vi "WS1050 36 DUT Characterization Ver1.0.vi"() -> ()   [LabVIEW 2012]
uses:
  WS_VCAP Driver 029/Source/WSVCAP Shell/Type Defs/WSVCAP SHL I2C DUT Mask Mode Enum.ctl
  <vilib>/Utility/file.llb/Read From Spreadsheet File (DBL).vi
panel:
  out "VISA resource name out":refnum<visa-resource-name>="GPIB0::3::INSTR"
  out "error out 2":errorcluster={"status"=TRUE, "code"=-63192, "source"="niLvFpga_Open_PXI-7813R.vi"}
  in  "Reg1_Bit Cntrl":string[](array[string])=["01", "02", "04", "08", "10", "20", "40", "80", "03", "06", "0C", "D8", "33", "66", "CC", "07", "0E", "1C", "38", "70", "E0", "0F", "1E", "3C", "78", "F0", "1F", "3E", "7C", "F8", "3F", "7E", "FC", "7F", "FE", "FD", "FB", "F7", "EF", "DF", "BF", "7F", "FC", "F9", "F3", "E7", "CF", "9F", "3F", "F8", "F1", "E3", "C7", "8F", "1F", "F0", "E1", "C3", "87", "0F", "E0", "C1", "83", "07", "C0", "81", "03", "AA", "55", "00"]
  out "date string":string="5/19/2014"
  out "PS1 Out":refnum<visa-resource-name>
  out "Ke2000 Out":refnum<visa-resource-name>="GPIB0::9::INSTR"
  in  "VPI_Cmd":string[](array[string])=["00", "3B", "00"]
  in  "VPI Name":string[](array[string])=["All_Drivers OFF", "All Drivers ON", "All Drivers OFF2"]
  in  "Tab Control":T1(tab)
  in  "No of Cmd":i64=3
  in  "Board#":string="BRD5"
  in  "Serial Number":string[][](table)=[["DUT", "SN"], ["DUT1", "1"], ["DUT2", "2"], ["DUT3", "3"], ["DUT4", "4"], ["DUT5", "5"], ["DUT6", "6"], ["DUT7", "7"], ["DUT8", "8"], ["DUT9", "9"], ["DUT10", "10"], ["DUT11", "11"], ["DUT12", "12"], ["DUT13", "13"], ["DUT14", "14"], ["DUT15", "15"], ["DUT16", "16"], ["DUT17", "17"], ["DUT18", "18"], ["DUT19", "19"], ["DUT20", "20"], ["DUT21", "21"], ["DUT22", "22"], ["DUT23", "23"], ["DUT24", "24"], ["DUT25", "25"], ["DUT26", "26"], ["DUT27", "27"], ["DUT28", "28"], ["DUT29", "29"], ["DUT30", "30"], ["DUT31", "31"], ["DUT32", "32"], ["DUT33", "33"], ["DUT34", "34"], ["DUT35", "35"], ["DUT36", "36"]]
  in  "SPI Clock Rate (Hz)":dbl=5000000.0 caption="Cycle Speed" format="%.1p Hz"
  in  "Wafer#":string="T7-EB"
  in  "File Name":string="CYC_WS1050_T7_EB_65C_40V_25DC_EMPTY_BRD5_141017_1"
  in  "TMN DC\\CAP Data Log File Path":path=path "C:/WS1050 36 DUT Data"
  in  "Test Program":string="WS1050 36 DUT Characterization Ver1.0"
  out "Current Date":string="8/28/2014"
  out "Current Time":string="0950"
  in  "Start Date":string="10/21/2014"
  in  "Start Time":string="1542"
  in  "Comment":string="CYC65C40V"
  in  "OK Button":bool
  in  "Calibration":bool
  in  "Verify CP":bool
  in  "CP Setting":i32(ring) items=["CP OFF", "CP ON", "CP 35V", "CP 40V", "DVA ON", "DVA OFF", "REG1 ON", "REG1 OFF", "REG2 ON", "REG2 OFF", "REG3 ON", "REG3 OFF"]
  in  "Stop Calibration":bool
  in  "Set VDD":dbl=3.3 format="%.3g"
  in  "Command":string[](array[string])=["07020100003B", "070201003B00", "0702013B0000"]
  in  "Clock Rate (Hz)":dbl=1000000.0 caption="Meas Speed" format="%.1p Hz"
  out "AR  Measurent(Hz)":dbl
  in  "PS1 Source":refnum<visa-resource-name>="GPIB0::5::INSTR"
  in  "Ke2000":refnum<visa-resource-name>="GPIB0::9::INSTR"
  in  "Set CP to Meas":i32(ring) items=["CP OFF", "CP 23.75V ", "CP 24.5V", "CP 25.25V", "CP 26V", "CP 26.75V", "CP 27.5V", "CP 28.25V", "CP 29V", "CP 29.75V", "CP 30.5V", "CP 31.25V", "CP 32V", "CP 32.75V", "CP 33.5V", "CP 34.25V", "CP 35V", "CP 35.75V", "CP 36.5V", "CP 37.25V", "CP 38V", "CP 38.75V", "CP 39.5V", "CP 40.25V", "CP 41V", "CP 41.75V", "CP 42.5V", "CP 43.25V", "CP 44V", "CP 50V", "CP 55V"]
  out "Simulate FPGA":bool
  out "Online":bool
  out "AR Cycling(Hz)":dbl=5000000.0
  in  "Ke2400":refnum<visa-resource-name>="GPIB0::3::INSTR"
  in  "Initialize AD7747":bool
  in  "DUT Mask Mode":T2=enum."All"
  in  "RFFE Slave Address":u8=7 caption="Slave Address" format="0x%02x"
  out "Activity Log":string="05/19/2014 -- 12:24:35.853::WSVCAP::APP::Application Started\n05/19/2014 -- 12:24:37.606::WSVCAP::WSVCAP SHL::WR I2C-REG:0x0A;MASK:0xFFFFFFFFFFFF;C1 DATA:22:22:22:22:22:22:22:22:22:22:22:22:22:22:22:22;C2 DATA:22:22:22:22:22:22:22:22:22:22:22:22:22:22:22:22;C3 DATA:22:22:22:22:22:22:22:22:22:22:22:22:22:22:22:22\r\n05/19/2014 -- 12:24:37.773::WSVCAP::WSVCAP SHL::WR I2C-ST:0,0,4,1\r\n05/19/2014 -- 12:24:37.903::WSVCAP::WSVCAP SHL::RD I2C-BYTES:4;ADD:0x00;MASK:0xFFFFFFFFFFFF\r\n05/19/2014 -- 12:24:38.045::WSVCAP::WSVCAP SHL::RD I2C:C1 DATA:2:2:2:2:2:2:2:2:2:2:2:2:2:2:2:2|A7:A9:AA:82:82:7F:82:81:82:81:83:82:81:82:82:81|46:36:BB:88:44:A3:E9:2B:32:20:ED:25:BB:3D:68:B|2C:6A:EB:A7:22:56:FE:CC:36:82:D7:B0:3B:48:F9:CC;C2 DATA:2:2:2:2:2:2:2:2:2:2:2:2:2:2:2:2|94:94:94:80:80:80:80:80:81:7E:7E:81:80:7E:80:80|47:33:15:82:62:B:E8:1C:D7:C3:7D:41:7C:B7:4C:2A|C4:B4:AE:8:1E:D1:4E:37:11:C0:6F:63:42:9D:63:B5;C3 DATA:2:2:2:2:2:2:2:2:2:2:2:2:2:2:2:2|95:95:95:81:81:7E:81:80:84:7D:80:83:81:7E:7F:80|AB:C4:14:B5:7B:52:DF:C9:79:5D:5F:30:99:31:1E:F4|6E:5C:F7:A8:C3:EB:7B:EF:33:92:89:77:4D:67:75:DD;STATUS:0:0:4:0\r\n05/19/2014 -- 12:24:38.046::WSVCAP::WSVCAP SHL::WR I2C-REG:0x0A;MASK:0xFFFFFFFFFFFF;C1 DATA:22:22:22:22:22:22:22:22:22:22:22:22:22:22:22:22;C2 DATA:22:22:22:22:22:22:22:22:22:22:22:22:22:22:22:22;C3 DATA:22:22:22:22:22:22:22:22:22:22:22:22:22:22:22:22\r\n05/19/2014 -- 12:24:38.089::WSVCAP::WSVCAP SHL::WR I2C-ST:0,0,4,1\r\n05/19/2014 -- 12:24:38.219::WSVCAP::WSVCAP SHL::RD I2C-BYTES:4;ADD:0x00;MASK:0xFFFFFFFFFFFF\r\n05/19/2014 -- 12:24:38.362::WSVCAP::WSVCAP SHL::RD I2C:C1 DATA:2:2:2:2:2:2:2:2:2:2:2:2:2:2:2:2|A7:AB:AA:82:82:82:83:83:82:82:82:82:7F:82:82:81|4B:32:96:83:3E:61:43:17:25:62:AB:4D:A2:40:2E:5|3C:76:2B:B4:EE:E4:A9:1A:AA:A:26:C7:21:2E:87:5B;C2 DATA:2:2:2:2:2:2:2:2:2:2:2:2:2:2:2:2|94:94:94:80:80:80:80:80:80:7F:80:81:80:80:7F:80|4A:32:19:7D:19:6C:79:46:61:7F:4B:B8:A5:30:F3:14|B4:70:A:8C:9C:DC:43:FA:1E:A:C6:21:A:A9:13:F3;C3 DATA:2:2:2:2:2:2:2:2:2:2:2:2:2:2:2:2|95:97:94:81:80:81:82:81:80:7E:81:84:7F:81:80:80|B2:32:D0:A7:9E:4C:AB:D4:EE:D9:F0:82:B7:91:7:FF|C1:91:B6:3D:D8:E:1B:4F:9F:6A:F1:6C:E7:3F:7:BA;STATUS:0:0:4:0\r\n05/19/2014 -- 12:24:38.364::WSVCAP::WSVCAP SHL::WR I2C-REG:0x0A;MASK:0xFFFFFFFFFFFF;C1 DATA:22:22:22:22:22:22:22:22:22:22:22:22:22:22:22:22;C2 DATA:22:22:22:22:22:22:22:22:22:22:22:22:22:22:22:22;C3 DATA:22:22:22:22:22:22:22:22:22:22:22:22:22:22:22:22\r\n05/19/2014 -- 12:24:38.406::WSVCAP::WSVCAP SHL::WR I2C-ST:0,0,4,1\r\n05/19/2014 -- 12:24:38.536::WSVCAP::WSVCAP SHL::RD I2C-BYTES:4;ADD:0x00;MASK:0xFFFFFFFFFFFF\r\n05/19/2014 -- 12:24:38.678::WSVCAP::WSVCAP SHL::RD I2C:C1 DATA:2:2:2:2:2:2:2:2:2:2:2:2:2:2:2:2|A7:A9:AB:82:82:81:82:82:82:82:82:82:82:82:82:81|46:71:4C:87:43:3D:7F:FC:25:4F:8E:54:97:3E:60:8C|AA:F4:1F:B5:CE:43:1F:36:9:87:9C:78:86:5:B6:8E;C2 DATA:2:2:2:2:2:2:2:2:2:2:2:2:2:2:2:2|94:94:94:80:7F:7F:80:80:80:80:80:81:80:80:80:80|49:36:18:7D:6E:C5:E4:3C:81:2E:41:D3:75:71:E3:72|E8:D3:E6:D1:E0:48:AE:D4:54:D:E8:8E:B4:41:68:4;C3 DATA:2:2:2:2:2:2:2:2:2:2:2:2:2:2:2:2|95:95:95:81:7F:7F:81:81:81:81:81:84:81:81:82:81|B3:F5:90:AB:82:69:7B:93:D0:77:E8:D5:E8:8C:84:E8|B9:AC:EE:2B:B6:71:8F:4A:74:31:56:BB:8A:B7:A0:C8;STATUS:0:0:4:0\r\n05/19/2014 -- 12:24:38.681::WSVCAP::WSVCAP SHL::WR I2C-REG:0x0A;MASK:0xFFFFFFFFFFFF;C1 DATA:22:22:22:22:22:22:22:22:22:22:22:22:22:22:22:22;C2 DATA:22:22:22:22:22:22:22:22:22:22:22:22:22:22:22:22;C3 DATA:22:22:22:22:22:22:22:22:22:22:22:22:22:22:22:22\r\n05/19/2014 -- 12:24:38.723::WSVCAP::WSVCAP SHL::WR I2C-ST:0,0,4,1\r\n05/19/2014 -- 12:24:38.854::WSVCAP::WSVCAP SHL::RD I2C-BYTES:4;ADD:0x00;MASK:0xFFFFFFFFFFFF\r\n05/19/2014 -- 12:24:38.996::WSVCAP::WSVCAP SHL::RD I2C:C1 DATA:2:2:2:2:2:2:2:2:2:2:2:2:2:2:2:2|A7:A9:AA:82:82:7F:83:81:82:81:84:82:7F:82:7F:82|43:FB:E:7F:3C:AD:35:35:26:A2:6C:21:4B:3D:8:6|63:9A:E1:F3:95:32:91:42:90:3C:78:1F:5C:D7:5F:D8;C2 DATA:2:2:2:2:2:2:2:2:2:2:2:2:2:2:2:2|94:94:94:80:80:80:80:80:81:80:7E:81:80:7E:7F:80|48:36:18:7F:5E:3D:69:83:DE:AE:A1:9E:31:AE:BB:96|15:A0:44:17:13:FD:CC:C8:6D:B2:EF:A7:C:C7:3B:F;C3 DATA:2:2:2:2:2:2:2:2:2:2:2:2:2:2:2:2|95:96:94:81:81:7E:82:80:84:80:80:84:7F:7E:7D:82|AD:3B:6D:A9:7C:57:9D:F5:7A:96:23:5C:36:2D:ED:5A|CD:46:DB:3B:C7:BD:70:60:33:B8:B:F7:63:A:51:4D;STATUS:0:0:4:0\r\n05/19/2014 -- 12:24:38.998::WSVCAP::WSVCAP SHL::WR I2C-REG:0x0A;MASK:0xFFFFFFFFFFFF;C1 DATA:22:22:22:22:22:22:22:22:22:22:22:22:22:22:22:22;C2 DATA:22:22:22:22:22:22:22:22:22:22:22:22:22:22:22:22;C3 DATA:22:22:22:22:22:22:22:22:22:22:22:22:22:22:22:22\r\n05/19/2014 -- 12:24:39.040::WSVCAP::WSVCAP SHL::WR I2C-ST:0,0,4,1\r\n05/19/2014 -- 12:24:39.170::WSVCAP::WSVCAP SHL::RD I2C-BYTES:4;ADD:0x00;MASK:0xFFFFFFFFFFFF\r\n05/19/2014 -- 12:24:39.311::WSVCAP::WSVCAP SHL::RD I2C:C1 DATA:2:2:2:2:2:2:2:2:2:2:2:2:2:2:2:2|A7:AA:AB:82:82:81:82:81:82:81:82:82:82:82:7F:82|44:F1:90:87:45:44:C8:2C:2C:F1:FC:1B:94:3B:3C:75|4A:49:95:19:99:73:64:3:23:24:F3:A2:5E:7F:C4:B6;C2 DATA:2:2:2:2:2:2:2:2:2:2:2:2:2:2:2:2|94:94:94:80:80:80:80:7F:80:80:7E:80:80:7E:7F:80|4C:36:17:7D:A8:9F:DE:C7:53:6D:8A:F4:41:A5:C6:E0|90:2E:24:C:D9:22:E4:76:3B:40:1D:53:33:B1:3E:4D;C3 DATA:2:2:2:2:2:2:2:2:2:2:2:2:2:2:2:2|95:97:95:81:81:7F:81:80:80:81:7F:82:81:7E:7D:82|AE:2B:A7:AB:CC:CD:A4:38:FD:17:80:F2:92:2D:45:C4|76:E5:D:B9:AD:B5:BA:8D:28:32:9E:42:B7:20:4A:D9;STATUS:0:0:4:0\r\n05/19/2014 -- 12:24:39.313::WSVCAP::WSVCAP SHL::WR I2C-REG:0x0A;MASK:0xFFFFFFFFFFFF;C1 DATA:22:22:22:22:22:22:22:22:22:22:22:22:22:22:22:22;C2 DATA:22:22:22:22:22:22:22:22:22:22:22:22:22:22:22:22;C3 DATA:22:22:22:22:22:22:22:22:22:22:22:22:22:22:22:22\r\n05/19/2014 -- 12:24:39.355::WSVCAP::WSVCAP SHL::WR I2C-ST:0,0,4,1\r\n05/19/2014 -- 12:24:39.486::WSVCAP::WSVCAP SHL::RD I2C-BYTES:4;ADD:0x00;MASK:0xFFFFFFFFFFFF\r\n05/19/2014 -- 12:24:39.628::WSVCAP::WSVCAP SHL::RD I2C:C1 DATA:2:2:2:2:2:2:2:2:2:2:2:2:2:2:2:2|A7:A9:AA:82:82:82:83:82:82:82:82:82:7F:82:7F:82|47:18:E4:87:3E:E7:6:65:25:92:37:38:A8:3E:89:85|7C:A7:7:2B:A3:7A:EC:EF:89:ED:F4:D3:D8:BC:3A:F5;C2 DATA:2:2:2:2:2:2:2:2:2:2:2:2:2:2:2:2|94:94:94:80:7F:80:80:7F:81:80:7E:80:80:80:81:80|49:37:17:80:76:25:6A:F8:DF:55:97:4D:B8:5B:2B:B1|13:E3:9A:3E:1A:2D:4F:B6:DB:E9:61:FA:8B:D6:9:CC;C3 DATA:2:2:2:2:2:2:2:2:2:2:2:2:2:2:2:2|95:95:95:81:7F:80:82:81:84:80:7F:81:80:81:7F:82|AF:93:3B:AF:5B:11:82:E4:7E:C3:2D:72:9:96:D9:A|DB:96:F2:10:5F:64:9A:C6:98:12:27:7D:10:D3:20:D9;STATUS:0:0:4:0\r\n05/19/2014 -- 12:24:40.132::WSVCAP::WSVCAP SHL::CLOSE\r\n"
  in  "C1 Cap DAC":u8=128 caption="B Data In" format="0x%02x"
  in  "C2 Cap DAC":u8=128 caption="B Data In" format="0x%02x"
  in  "C3 Cap DAC":u8=128 caption="B Data In" format="0x%02x"
  out "IDD Brd(uA)":string
  in  "CP to Meas":i32(ring)=1 items=["CP HDC 35V", "CP HDC 40.25V", "CP HDC 27.5V", "CP HDC 30.5V", "CP HDC 44V"]
  in  "CP VPI":i32(ring) items=["CP HDC 35V", "CP HDC 40.25V", "CP HDC 27.5V", "CP HDC 30.5V", "CP HDC 44V"]
  in  "Repeat Meas(s)":u32
  in  "Real No. From\nLookup Table":bool
  in  "Control Panel":T3={"C-V Sweep"=TRUE, "HD/CYC"=FALSE, "E-CAL"=FALSE, "DVA"=FALSE, "VPI"=FALSE, "VSA"=FALSE, "HS"=FALSE}
  out "C-V Sweep":bool
  out "HD/CYC":bool
  out "E-CAL":bool
  out "DVA":bool
  out "VPI":bool
  out "VSA":bool
  out "HS":bool
  in  "Lot#":string="WS1050"
  out "AD7747 Values":string[][](table)
  in  "Freq(Hz)":string="12K"
  in  "Reset P/S":bool
  in  "Test Sequences":i32(ring) items=["C1_C2_C3", "C2_C1_C3", "C3_C2_C1"]
  in  "WS1050/51":bool=TRUE
  in  "CP with DVA ON":i32(ring) items=["CP HDC 35V", "CP HDC 40.25V", "CP HDC 27.5V", "CP HDC 30.5V", "CP HDC 44V"]
  in  "% Duty Cycle":string="33"
  in  "Cmd To HD":string="0702013B3B3B"
  in  "Post CMd Delay":dbl[](array[numeric])=[1.8e-05, 1.8e-05, 1.8e-05] min=0.0 max=0.5 format="%#.0p s"
  in  "Cmin/Act":bool=TRUE
  out "40V_1":string[][](table)
  out "NOM IDD OFF(uA)":string
  out "40V_2":string[][](table)
  out "40V_3":string[][](table)
  out "Total Time":u64
  in  "Set HD/Cycle \nto Complete":u64=50000000000
  out "No of HD/Cycle\nCompleted":u64
  out "Cycle Count":u64 min=1 max=4 step=1
  out "Loop \ncompleted":i32=1
  out "Previous Time":string="12:20:26 PM"
  out "STATUS":string="Idle...."
  out "Total Delta C2(pF)":string[](array[string])
  out "Total Delta C1(pF)":string[](array[string])
  out "Total Delta C3(pF)":string[](array[string])
  out "RB Reg for HD":string[](array[string])
  out "RB Reg for HD/Cycle":string[](array[string])
  out "VPI C2":string[][](table)
  out "VPI C3":string[][](table)
  out "NOM IDD ON (uA)":string
  out "IDD_HD/CYC (uA)":string="164.601255E+0"
  in  "stop During HD/Cycles":bool
  in  "stop":bool
  out "IDD Stdby(uA)":string="2.606990E+0"
  out "VPI C1":string[][](table)
  out "Loops Run":u64
  out "CP Voltage":string
  out "VSA_V1":string[][](table)
  out "VSA_V2":string[][](table)
  out "VSA_V3":string[][](table)
  in  "VSA Voltage(V)":dbl[](array[numeric])=[-10.0, 0.0, 10.0]
  in  "DC_Temp":i32=65
  in  "HD/CYC Temp":i32=65
  in  "Time All ON (s)":u32=120
  in  "Time All OFF (s)":u32=120
  in  "HD_DC (Min)":u64=259200
  out "LPs Count":i32
  in  "X Repeat":i32=100
  out "No LPs to RP":i32
  out "Run Loops":i32=1
  out "TTCompleted":u64=2000
  in  "TTF Completed":u64=50000000000
  out "% Delta C_T0":string[][](array[string])
  out "% Delta C":string[][](array[string])
  out "EFuse RB T0":string[](array[string])
  out "Current EFuse Read back":string[](array[string])
  out "EFuse Readback Status":bool[](array[boolean])
  in  "DeltaC Target Setting(pF)":dbl=7.375
  out "error out":errorcluster
  in  "error in (no error)":errorcluster
  in  "HD RP":dbl=60.0
  in  "Cycle RP":dbl=10000.0
  out "Plot_1":dbl[][](graph) caption="(Y) Multi Plot 2"
  out "Plot_2":dbl[][](graph) caption="(Y) Multi Plot 2"
  out "Plot_3":dbl[][](graph) caption="(Y) Multi Plot 2"
  in  "Debug":bool
  in  "No of Rows\nFrom Spread Sheet":i32
  in  "Plot Delta Cmin":bool=TRUE
  in  "Plot":T4(ring)
  in  "Bank 2":i32(ring)=4 items=["C1", "C2", "C3", "D_C1", "D_C2", "D_C3"]
  in  "Bank":i32(ring)=3 items=["C1", "C2", "C3", "D_C1", "D_C2", "D_C3"]
  in  "Bank 3":i32(ring)=5 items=["C1", "C2", "C3", "D_C1", "D_C2", "D_C3"]
  # "Company:  WiSpry Inc\n20 Fairbanks Ste 198 Irvine CA 92618\n\nAuthor:  Andy V Tran\nCreated:  06/04/2015\nLabVIEW 2012 Pro\nTest Program:  WS1050 36 DUT Characterization Ver1.0\nFPGA: WS_VCAP Driver 029"
  # "Note for HD Duty Cycle:\n1.  Set time to start HD_DC (Min), default is 259200 (6 months) \n2.  Set Time for Duty Cycle ON/OFF, default setting is 2 minutes\n3.  No of Loops to RP = 3600s/(Time ALL ON(s) + Time ALL + OFF(s))\n4.  Set X Repeat = no of runs, default is 100 runs\n5.  Set TTF Completed to stop the test.\n\nVer 1.4 updated based on Ver1.3:\n1.  Updated P/S E3631A Driver\n2.  Updated KE2400 Driver"
  # "Minutes"
  # "X1000"
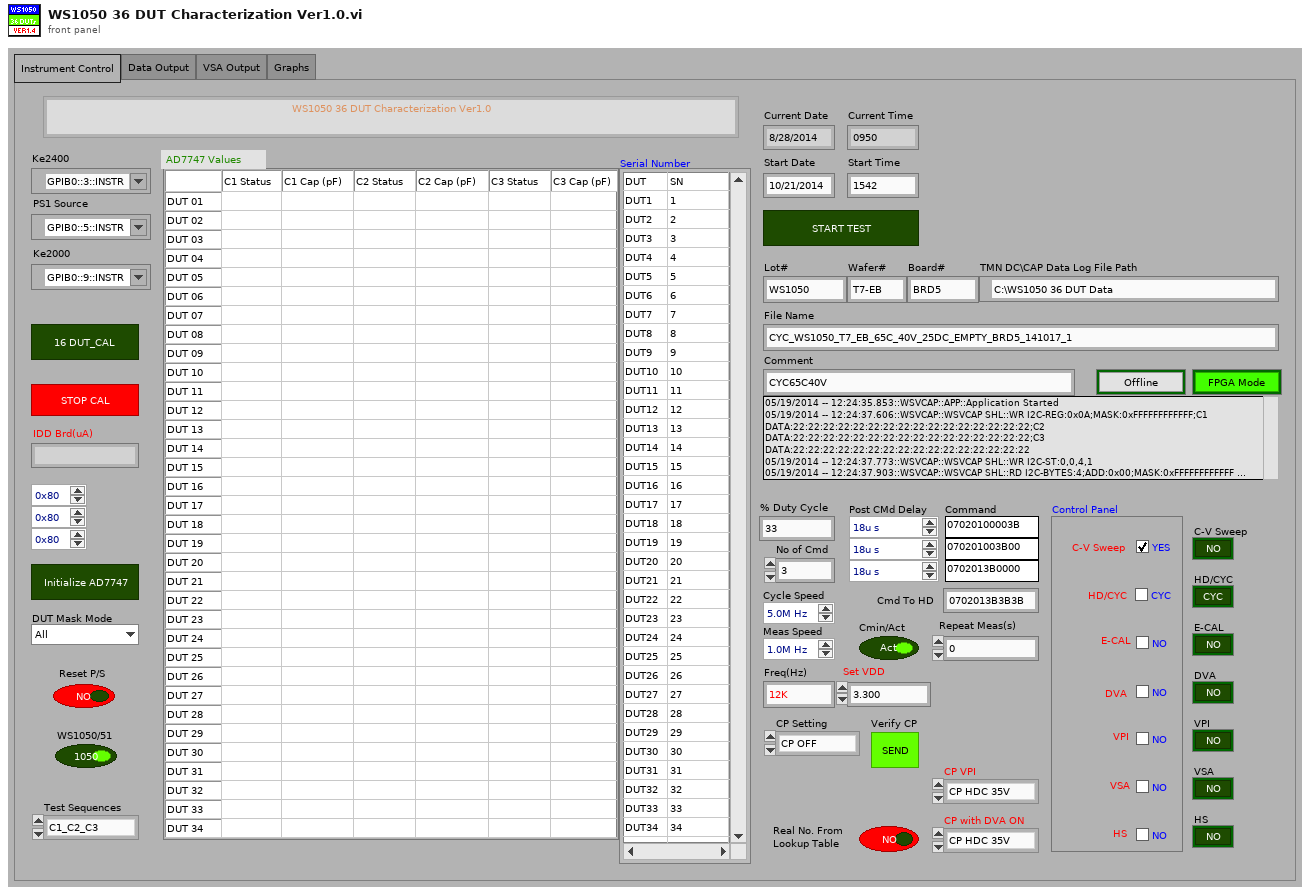
[diagram p1: front panel]
types:
  T1 = enum32{"Instrument Control", "Data Output", "VSA Output", "Graphs"}
  T2 = typedef "WSVCAP SHL I2C DUT Mask Mode Enum.ctl" = enum16{"Custom", "C1", "C2", "C3", "All"}
  T3 = cluster{"C-V Sweep":bool, "HD/CYC":bool, "E-CAL":bool, "DVA":bool, "VPI":bool, "VSA":bool, "HS":bool}
  T4 = enum16{"ALL DUTs", "DUT 01", "DUT 02", "DUT 03", "DUT 04", "DUT 05", "DUT 06", "DUT 07", "DUT 08", "DUT 09", "DUT 10", "DUT 11", "DUT 12", "DUT 13", "DUT 14", "DUT 15", "DUT 16", "DUT 17", "DUT 18", "DUT 19", "DUT 20", "DUT 21", "DUT 22", "DUT 23", "DUT 24", "DUT 25", "DUT 26", "DUT 27", "DUT 28", "DUT 29", "DUT 30", "DUT 31", "DUT 32", "DUT 33", "DUT 34", "DUT 35", "DUT 36"}
  T5 = typedef "WSVCAP SHL Core System Cluster.ctl" = cluster{"Settings":T6, "FPGA Resource":tag, "Online":bool, "I2C Wait Ticks":u32, "SPI Wait Ticks":u32, "RFFE Wait Ticks":u32}
  T6 = typedef "WSVCAP SHL I2C Settings Cluster.ctl" = cluster{"FPGA Resource Name":string, "I2C Slave Address":u8, "I2C Clock Rate (Hz)":dbl, "SPI Clock Rate (Hz)":dbl, "RFFE Slave Address":u8, "RFFE Clock Rate (Hz)":dbl, "Simulate FPGA":bool, "C1 Cap DAC Default":u8, "C2 Cap DAC Default":u8, "C3 Cap DAC Default":u8}
  T7 = enum16{"Idle...", "Voltage 1", "Voltage 2", "Voltage 3"}[]
  T8 = cluster{"Test Program ":string, "Comment":string, "Data Out":string, "Data Out":string, "CP Voltage":string, string, "Data Out":string, "CP Voltage":string, "string":string, "Freq(Hz)":string, "Board#":string}
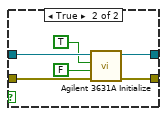
[diagram p2: hidden frame]
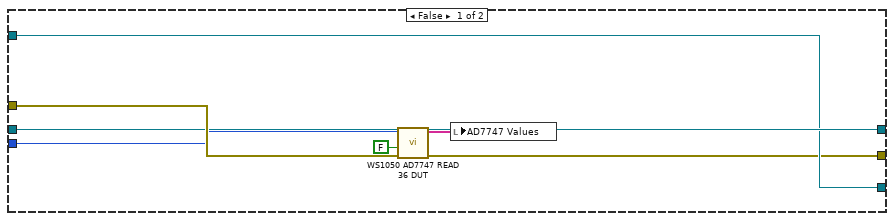
[diagram p10: hidden frame]
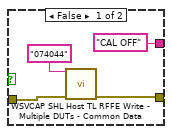
[diagram p11: hidden frame]
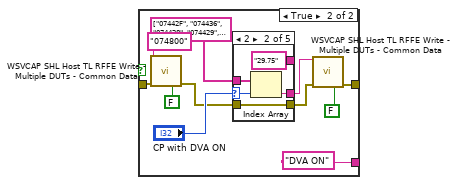
[diagram p12: hidden frame]
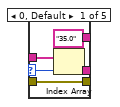
[diagram p13: hidden frame]
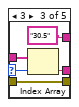
[diagram p14: hidden frame]
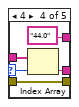
[diagram p15: hidden frame]
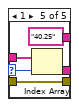
[diagram p16: hidden frame]
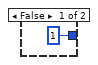
[diagram p17: hidden frame]
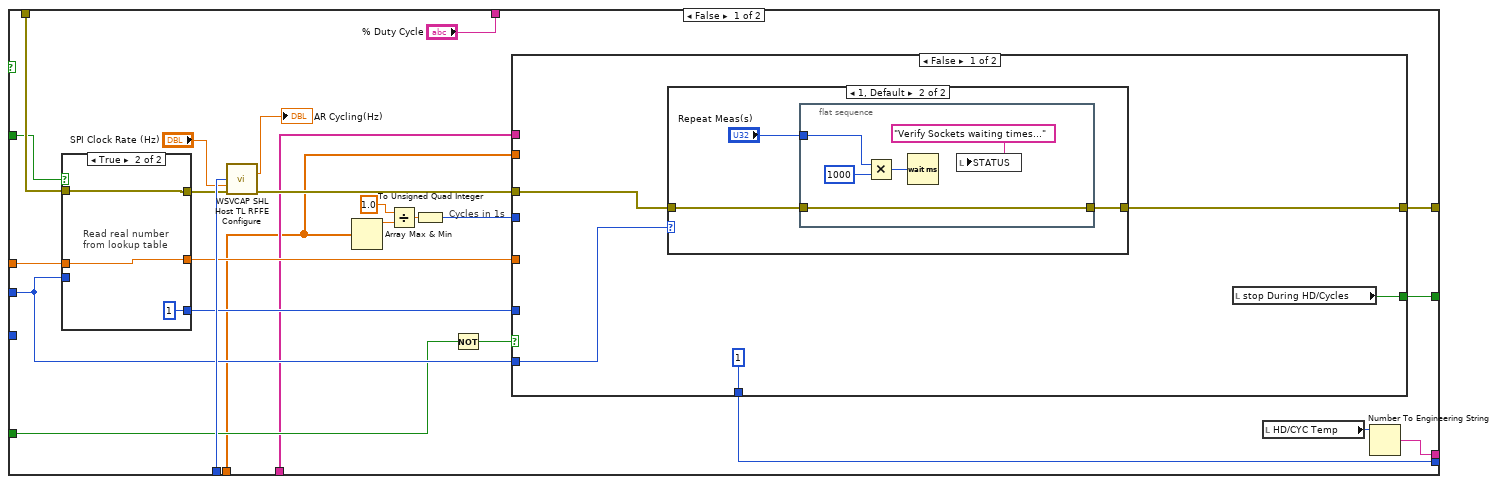
[diagram p18: hidden frame]
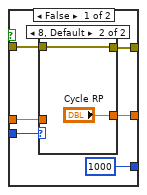
[diagram p19: hidden frame]
diagram:
  w19 = TRUE
  w25 = u16 0 items=["Off", "Moving Filter", "Repeating Filter"] ("Digital Filter (0: Off)")
  w26 = u16 7 items=["3.5 Digits"=4, "4.5 Digits"=5, "5.5 Digits"=6, "6.5 Digits"=7] ("Resolution (7: 6.5 digits)")
  n1 = case shown="True" w19 {
    tunnel: "error in (no error)" -> [w33 w34]
    tunnel: [w33 w41] -> w5
    frame False {
    }
    frame True {
      n2 = call "WSVCAP SHL Host TL Initialize.vi"("error in"=w34) -> ("error out"=w35:errorcluster)  [unwired: 13 in, 1 out]
      n3 = control-ref of="Activity Log"() -> (w37:refnum<vi>)
      n4 = call "ACT LG Activity Log Core.vi"("Display Ref"=w37, "Source"="WSVCAP", "Error In (no error)"=w35) -> ("Error Out"=w36:errorcluster)  [unwired: 11 in, 1 out]
      n5 = call "WSVCAP SHL Host TL Status Manager.vi"("error in"=w36) -> ("System Out"=w42:T5, "error out"=w41:errorcluster)  [unwired: 13 in]
      n6 = Unbundle By Name(w42) -> ("Online"=→"Online":bool, "Settings.Simulate FPGA"=→"Simulate FPGA":bool)
    }
  }
  n7 = case shown="True" TRUE {
    tunnel: w5 -> [w43 w48]
    tunnel: [w44 w47] -> w16
    tunnel: [w43 w46] -> w9
    tunnel: "Ke2400" -> [w44 w45]
    frame False {
    }
    frame True {
      n8 = VISA Write(VISA resource name=w45, write buffer="SOUR:FUNC VOLT;VOLT:MODE FIX;RANG 100;LEV 0.0;:SENS:FUNC \"CURR\";CURR:PROT 60E-3;RANG 100E-3;:OUTP ON", error in (no error)=w48) -> (VISA resource name out=w47:refnum<visa-resource-name>, error out=w46:errorcluster)  [unwired: 1 out]
    }
  }
  n9 = case shown="False" "Reset P/S" {
    tunnel: "PS1 Source" -> [w50 w57]
    tunnel: [w50 w55] -> w30
    tunnel: w5 -> [w51 w53]
    tunnel: [w51 w52] -> w4
    frame False {
    }
    frame True {
      n10 = call "Agilent 3631A Initialize.vi"("error in (no error)"=w53, "Default"=FALSE ("Reset? (T: Yes)"), "Reset"=TRUE ("ID Query? (T: Yes)"), "VISA resource name"=w57) -> ("error out"=w52:errorcluster, "VISA resource name out"=w55:refnum<visa-resource-name>)  [unwired: 6 in]
    }
  }
  n11 = call "Ke2000 Initialize.vi"("error in (no error)"=w5, "VISA resource name"="Ke2000") -> ("error out"=w27:errorcluster, "VISA resource name out"=w28:refnum<visa-resource-name>)  [unwired: 8 in]
  n12 = call "Ke2000 Configure DC Current.vi"("Resolution (7: 6.5 digits)"=w26, "Digital Filter (0: Off)"=w25, "Auto Range? (T: Auto)"=FALSE, "error in (no error)"=w27, "Custom Range (0 A)"=1.0, "VISA resource name"=w28) -> ("error out"=w6:errorcluster, "VISA resource name out"=w23:refnum<visa-resource-name>)  [unwired: 4 in]
  n13 = case shown="True" TRUE {
    tunnel: [_ w58] -> w32
    frame False {
    }
    frame True {
      n14 = call-poly <vilib>:"Read From Spreadsheet File.vi"("number of rows (all:-1)"=-1) -> ("all rows"=w58:dbl[][])  [unwired: 6 in, 4 out]
    }
  }
  n15 = Merge Errors(w9, w6, w4) -> (w17:errorcluster)
  n16 = while {
    tunnel: w17 -> [w62]
    tunnel: [w71] -> w13
    tunnel: w32 -> [w87]
    tunnel: w30 -> [w75]
    tunnel: w23 -> [w76]
    tunnel: [w85] -> w22
    tunnel: [w84] -> w21
    tunnel: w16 -> [w82]
    tunnel: [w81] -> w14
    tunnel: [FALSE ("stop")] -> w7
    i -> [w83]
    stop <- w88 stop-if-true
    n17 = case shown="0" w83 {
      tunnel: w62 -> [w99 w101]
      tunnel: [w98 w101] -> w78
      tunnel: "RFFE Slave Address" -> [w96 _]
      frame 0 {
        w92 = dbl[][] []
        w91 = "" ("uA")
        w93 = string[][] []
        w94 = string[] [] ("EFuse Read back")
        w100 = u64 0 ("No of HD/Cycle\nCompleted")
        n18 = local write "RB Reg for HD/Cycle"(w94) -> ()
        n19 = local write "Current EFuse Read back"(w94) -> ()
        n20 = local write "EFuse RB T0"(w94) -> ()
        n21 = local write "Total Delta C1(pF)"(w94) -> ()
        n22 = local write "Total Delta C2(pF)"(w94) -> ()
        n23 = local write "Total Delta C3(pF)"(w94) -> ()
        n24 = local write "No of HD/Cycle\nCompleted"(w100) -> ()
        n25 = local write "Cycle Count"(w100) -> ()
        n26 = local write "VPI C2"(w93) -> ()
        n27 = local write "VSA_V3"(w93) -> ()
        n28 = local write "VSA_V1"(w93) -> ()
        n29 = local write "40V_2"(w93) -> ()
        n30 = local write "40V_1"(w93) -> ()
        n31 = local write "NOM IDD OFF(uA)"(w91) -> ()
        n32 = local write "NOM IDD ON (uA)"(w91) -> ()
        n33 = local write "IDD Brd(uA)"(w91) -> ()
        n34 = local write "VSA_V2"(w93) -> ()
        n35 = local write "VPI C1"(w93) -> ()
        n36 = local write "VPI C3"(w93) -> ()
        n37 = local write "% Delta C"(w93) -> ()
        n38 = local write "% Delta C_T0"(w93) -> ()
        n39 = local write "40V_3"(w93) -> ()
        n40 = call "WSVCAP SHL Host TL RFFE Configure.vi"("RFFE Slave Address"=w96, "Clock Rate (Hz)"="Clock Rate (Hz)", "error in"=w99) -> ("Actual Rate (Hz)"=→"AR  Measurent(Hz)":dbl, "error out"=w98:errorcluster)  [unwired: 11 in]
        n41 = local write "Plot_3"(w92) -> ()
        n42 = local write "Plot_1"(w92) -> ()
        n43 = local write "Plot_2"(w92) -> ()
      }
      frame 1, Default {
      }
    }
    n44 = while {
      tunnel: ["stop"] -> w80
      tunnel: w78 -> [w127]
      tunnel: [w119] -> w72
      tunnel: w75 -> [w126]
      tunnel: w76 -> [w121]
      tunnel: [w122] -> w74
      tunnel: [w120] -> w73
      tunnel: [w117] -> w69
      tunnel: [w116] -> w68
      tunnel: [w115] -> w67
      tunnel: [w114] -> w66
      tunnel: [w113] -> w65
      tunnel: [w112] -> w64
      tunnel: [w111] -> w63
      tunnel: ["Command"] -> w61
      tunnel: ["Post CMd Delay"] -> w60
      stop <- w134 stop-if-true
      # "Set Date & Time to Start Test"
      n45 = case shown="True" "Initialize AD7747" {
        tunnel: w127 -> [w143 w148]
        tunnel: [w143 w144] -> w110
        tunnel: w126 -> [w142 w146]
        tunnel: [w142 w145] -> w125
        frame False {
        }
        frame True {
          w149 = T7 [enum."Voltage 2", enum."Voltage 3", enum."Voltage 1"] items=["Idle...", "Voltage 1", "Voltage 2", "Voltage 3"]
          n46 = for {
            tunnel: w146 -> [w159]
            tunnel: w149 -> [w157] mode=indexing
            tunnel: [w156] -> w145
            shift-right: [w152] -> w147
            shift-left: w148 -> [w160]
            n47 = local read "Set VDD"() -> (w155:dbl)
            n48 = call "E3631A_Voltage Controller updated.vi"("VISA resource name"=w159, "I_VDD(A)"=0.5, "Channel Controller"=w157, "Voltage 1"=w155, "Voltage 2"=3.3, "error in (no error)"=w160, "I_3.3V (A)"=0.5) -> ("VISA resource name out"=w156:refnum<visa-resource-name>, "error out"=w151:errorcluster)  [unwired: 7 in]
            n49 = call "Delay T4.vi"("milliseconds to wait"=u32 100, "error in (no error)"=w151) -> ("error out"=w152:errorcluster)  [unwired: 9 in]
          }
          n50 = call "WS1050_AD7747_Init 36DUT.vi"("error in"=w147) -> ("error out"=w144:errorcluster)  [unwired: 10 in]
        }
      }
      n51 = call "Time_stamp.vi"() -> ("date/time string"=w139:string, "date string"=w141:string)  [unwired: 2 in]
      "Current Date" <- w141
      "Current Time" <- w139
      n52 = Equal?(x=w141, y="Start Date") -> (x = y?=w137:bool)
      n53 = Equal?(x=w139, y="Start Time") -> (x = y?=w136:bool)
      n54 = And(x=w137, y=w136) -> (x .and. y?=w133:bool)
      n55 = Compound Arithmetic op=OR(w133, "OK Button", "stop") -> (w134:bool)
      n56 = case shown="True" "Calibration" {
        tunnel: w110 -> [w190 w207]
        tunnel: [w184 w204] -> w108
        tunnel: w125 -> [w189 w203]
        tunnel: "DUT Mask Mode" -> [w188 w199]
        tunnel: [w189 w198] -> w123
        tunnel: w121 -> [w187 w194]
        tunnel: [w187 w191] -> w120
        frame False {
          n57 = call "WS1050 AD7747 READ 36 DUT.vi"("error in"=w190, "Log (T)"=FALSE, "DUT Mask Mode (All)"=w188) -> ("error out"=w184:errorcluster, "AD7747 Values"=w185:string[][])  [unwired: 7 in]
          n58 = local write "AD7747 Values"(w185) -> ()
        }
        frame True {
          n59 = flat-sequence {
            tunnel: w207 -> [w216]
            tunnel: [w211] -> w206
            tunnel: w203 -> [w215]
            tunnel: [w214] -> w202
            tunnel: w199 -> [w213]
            tunnel: [w213] -> w200
            tunnel: w194 -> [w209]
            tunnel: [w208] -> w193
            tunnel: w206 -> [w240]
            tunnel: [w239] -> w205
            tunnel: w202 -> [w238]
            tunnel: [w238] -> w201
            tunnel: w200 -> [w237]
            tunnel: "C1 Cap DAC" -> [w233]
            tunnel: "C2 Cap DAC" -> [w232]
            tunnel: "C3 Cap DAC" -> [w231]
            tunnel: w193 -> [w230]
            tunnel: [w230] -> w192
            tunnel: w205 -> [w249]
            tunnel: [w252] -> w204
            tunnel: w201 -> [w251]
            tunnel: [w248] -> w198
            tunnel: w192 -> [w247]
            tunnel: [w247] -> w191
            frame #0 {
              w217 = T7 [enum."Voltage 2", enum."Voltage 3", enum."Voltage 1"] items=["Idle...", "Voltage 1", "Voltage 2", "Voltage 3"]
              n60 = for {
                tunnel: w215 -> [w228]
                tunnel: w217 -> [w226] mode=indexing
                tunnel: [w225] -> w214
                shift-right: [w223] -> w210
                shift-left: w216 -> [w229]
                n61 = local read "Set VDD"() -> (w220:dbl)
                n62 = call "E3631A_Voltage Controller updated.vi"("VISA resource name"=w228, "I_VDD(A)"=0.5, "Channel Controller"=w226, "Voltage 1"=w220, "Voltage 2"=3.3, "error in (no error)"=w229, "I_3.3V (A)"=0.5) -> ("VISA resource name out"=w225:refnum<visa-resource-name>, "error out"=w222:errorcluster)  [unwired: 7 in]
                n63 = call "Delay T4.vi"("milliseconds to wait"=u32 100, "error in (no error)"=w222) -> ("error out"=w223:errorcluster)  [unwired: 9 in]
              }
              n64 = call "Ke2000 Single Reading.vi"("error in (no error)"=w210, "VISA resource name"=w209) -> ("error out"=w211:errorcluster, "VISA resource name out"=w208:refnum<visa-resource-name>, "uA"=→"IDD Brd(uA)":string)  [unwired: 5 in, 2 out]
              n65 = One Button Dialog(message="Please verify all sockets should be empty...") -> ()  [unwired: 1 in, 1 out]
            }
            frame #1 {
              n66 = call "WS1050 CAPDAC Setting.vi"("DUT Mask Mode (All)"=w237, "error in"=w240, "C3 Cap DAC"=w231, "C2 Cap DAC"=w232, "C1 Cap DAC"=w233) -> ("error out"=w235:errorcluster)  [unwired: 5 in, 1 out]
              n67 = call "WS1050 OFFSET CAL.vi"("error in"=w235, "OFFSET CAL"=TRUE ("Read?")) -> ("error out"=w234:errorcluster)  [unwired: 8 in, 1 out]
              n68 = while {
                tunnel: w234 -> [w246]
                tunnel: [w245] -> w239
                tunnel: w237 -> [w243]
                stop <- "Stop Calibration" stop-if-true
                n69 = call "WS1050 AD7747 READ 36 DUT.vi"("error in"=w246, "Log (T)"=FALSE, "DUT Mask Mode (All)"=w243) -> ("error out"=w245:errorcluster, "AD7747 Values"=→"AD7747 Values":string[][])  [unwired: 7 in]
              }
            }
            frame #2 {
              w250 = T7 [enum."Voltage 2", enum."Voltage 3", enum."Voltage 1"] items=["Idle...", "Voltage 1", "Voltage 2", "Voltage 3"]
              n70 = for {
                tunnel: w251 -> [w264]
                tunnel: w250 -> [w261] mode=indexing
                tunnel: [w260] -> w248
                shift-right: [w256] -> w252
                shift-left: w249 -> [w262]
                n71 = call "E3631A_Voltage Controller updated.vi"("VISA resource name"=w264, "I_VDD(A)"=0.5, "Channel Controller"=w261, "Voltage 1"=0.0, "Voltage 2"=3.3, "error in (no error)"=w262, "I_3.3V (A)"=0.5) -> ("VISA resource name out"=w260:refnum<visa-resource-name>, "error out"=w255:errorcluster)  [unwired: 7 in]
                n72 = call "Delay T4.vi"("milliseconds to wait"=u32 100, "error in (no error)"=w255) -> ("error out"=w256:errorcluster)  [unwired: 9 in]
              }
              n73 = One Button Dialog(message="Calibration Completed....") -> ()  [unwired: 1 in, 1 out]
            }
          }
        }
      }
      n74 = call "Control Panel.vi"("error in (no error)"=w110, "Control Panel"="Control Panel") -> ("error out"=w107:errorcluster, "VPI"=w113:bool, "DVA"=w114:bool, "E-CAL"=w115:bool, "VSA"=w112:bool, "HD/CYC"=w116:bool, "HS"=w111:bool, "Verify Socket"=w117:bool)  [unwired: 2 in]
      "C-V Sweep" <- w117
      "E-CAL" <- w115
      "VPI" <- w113
      "VSA" <- w112
      "HS" <- w111
      "HD/CYC" <- w116
      "DVA" <- w114
      n75 = Merge Errors(w107, w108) -> (w109:errorcluster)
      n76 = case shown="True" "Verify CP" {
        tunnel: [w161 w165] -> w119
        tunnel: w123 -> [w162 w168]
        tunnel: [w162 w166] -> w122
        tunnel: w109 -> [w161 w164]
        frame False {
        }
        frame True {
          w169 = T7 [enum."Voltage 2", enum."Voltage 3", enum."Voltage 1"] items=["Idle...", "Voltage 1", "Voltage 2", "Voltage 3"]
          # "Verify CP"
          n77 = for {
            tunnel: w168 -> [w182]
            tunnel: w169 -> [w180] mode=indexing
            shift-right: [w177] -> w167
            shift-left: w164 -> [w183]
            tunnel: [w175] -> w166
            n78 = local read "Set VDD"() -> (w179:dbl)
            n79 = call "E3631A_Voltage Controller updated.vi"("VISA resource name"=w182, "I_VDD(A)"=0.5, "Channel Controller"=w180, "Voltage 1"=w179, "Voltage 2"=3.3, "error in (no error)"=w183, "I_3.3V (A)"=0.5) -> ("VISA resource name out"=w175:refnum<visa-resource-name>, "error out"=w178:errorcluster)  [unwired: 7 in]
            n80 = call "Delay T4.vi"("milliseconds to wait"=u32 100, "error in (no error)"=w178) -> ("error out"=w177:errorcluster)  [unwired: 9 in]
          }
          n81 = Index Array(array=string[] ["074000", "074040", "07476F", "074776", "074800", "074820", "07413B", "074100", "07423B", "074200", "07433B", "074300"], index="CP Setting") -> (element=w170:string)
          n82 = call "WSVCAP SHL Host TL RFFE Write - Multiple DUTs - Common Data.vi"("Data Out"=w170, "error in"=w167, "Log (T)"=FALSE) -> ("error out"=w165:errorcluster)  [unwired: 12 in]
        }
      }
      n83 = Array Subset(array="Post CMd Delay", length="No of Cmd") -> (w105:dbl[])  [unwired: 1 in]
      n84 = Array Subset(array="Command", length="No of Cmd") -> (w106:string[])  [unwired: 1 in]
      n85 = property on="Post CMd Delay" class="Arr (strict)"("Number of Rows"="No of Cmd") -> ()  [unwired: 2 in, 2 out]
      n86 = local write "Command"(w106) -> ()
      n87 = local write "Post CMd Delay"(w105) -> ()
      n88 = property on="Command" class="Arr (strict)"("Number of Rows"="No of Cmd") -> ()  [unwired: 2 in, 2 out]
      n89 = Wait Until Next ms Multiple(millisecond multiple=u32 100) -> ()  [unwired: 1 out]
    }
    n90 = case shown="False" w80 {
      tunnel: w72 -> [w324 w1837]
      tunnel: [w309 w1837] -> w71
      tunnel: w87 -> [w325 _]
      tunnel: w74 -> [w323 w1835]
      tunnel: w73 -> [w315 w1836]
      tunnel: [w321 w1836] -> w85
      tunnel: [w319 w1835] -> w84
      tunnel: w82 -> [w312 w1834]
      tunnel: [w308 w1834] -> w81
      tunnel: "RFFE Slave Address" -> [w303 _]
      tunnel: [FALSE ("stop During HD/Cycles") FALSE ("stop During HD/Cycles")] -> w70
      tunnel: w69 -> [w278 _]
      tunnel: w68 -> [w277 _]
      tunnel: w67 -> [w276 _]
      tunnel: w66 -> [w275 _]
      tunnel: w65 -> [w274 _]
      tunnel: w64 -> [w273 _]
      tunnel: w63 -> [w272 _]
      tunnel: w61 -> [w266 _]
      tunnel: w60 -> [w265 _]
      frame False {
        w304 = u64 0 ("Total Completed")
        w283 = u32 100 ("milliseconds to wait")
        w320 = T7 [enum."Voltage 2", enum."Voltage 3", enum."Voltage 1"] items=["Idle...", "Voltage 1", "Voltage 2", "Voltage 3"]
        w322 = T7 [enum."Voltage 2", enum."Voltage 3", enum."Voltage 1"] items=["Idle...", "Voltage 1", "Voltage 2", "Voltage 3"]
        # "VSA"
        # "HS"
        # "HD/CYC"
        # "DVA"
        # "E-CAL"
        # "VPI"
        # "Verify Socket"
        n91 = for {
          tunnel: w324 -> [w1832]
          tunnel: w323 -> [w1831]
          tunnel: w322 -> [w1829] mode=indexing
          tunnel: [w1824] -> w317
          tunnel: [w1828] -> w307
          n92 = local read "Set VDD"() -> (w1827:dbl)
          n93 = call "E3631A_Voltage Controller updated.vi"("VISA resource name"=w1831, "I_VDD(A)"=0.5, "Channel Controller"=w1829, "Voltage 1"=w1827, "Voltage 2"=3.3, "error in (no error)"=w1832, "I_3.3V (A)"=0.5) -> ("VISA resource name out"=w1828:refnum<visa-resource-name>, "error out"=w1825:errorcluster)  [unwired: 7 in]
          n94 = call "Delay T4.vi"("milliseconds to wait"=u32 100, "error in (no error)"=w1825) -> ("error out"=w1824:errorcluster)  [unwired: 9 in]
        }
        n95 = local write "Total Time"(w304) -> ()
        n96 = local write "TTCompleted"(w304) -> ()
        n97 = call "WSVCAP SHL Host TL RFFE Write - Multiple DUTs - Common Data.vi"("Data Out"="074000", "error in"=w317, "Log (T)"=FALSE) -> ("error out"=w318:errorcluster)  [unwired: 12 in]
        n98 = local read "IDD Brd(uA)"() -> (w292:string)
        n99 = call "Delay T4.vi"("milliseconds to wait"=w283, "error in (no error)"=w318) -> ("error out"=w316:errorcluster)  [unwired: 9 in]
        n100 = call "Ke2000 Single Reading.vi"("error in (no error)"=w316, "VISA resource name"=w315) -> ("error out"=w293:errorcluster, "VISA resource name out"=w314:refnum<visa-resource-name>, "uA"=w295:string)  [unwired: 5 in, 2 out]
        n101 = call "Substration.vi"("error in (no error)"=w293, "Input2"=w292, "Input1"=w295) -> ("error out"=w268:errorcluster, "In1 - In2"=w294:string)  [unwired: 7 in]
        "IDD Stdby(uA)" <- w294
        n102 = case shown="True" w277 {
          tunnel: [1 ("X Repeat") w386] -> w306
          frame False {
          }
          frame True {
            n103 = local read "X Repeat"() -> (w386:i32)
          }
        }
        n104 = call "WSVCAP SHL Host TL RFFE Write - Multiple DUTs - Common Data.vi"("Data Out"="074040", "error in"=w268, "Log (T)"=FALSE) -> ("error out"=w267:errorcluster)  [unwired: 12 in]
        n105 = call "Delay T4.vi"("milliseconds to wait"=w283, "error in (no error)"=w267) -> ("error out"=w301:errorcluster)  [unwired: 9 in]
        n106 = case shown="False" w275 {
          tunnel: w301 -> [w348 w357]
          tunnel: [w347 w355] -> w299
          tunnel: ["DVA OFF" ("Data Out") "DVA ON" ("Data Out")] -> w300
          frame False {
            n107 = call "WSVCAP SHL Host TL RFFE Write - Multiple DUTs - Common Data.vi"("Data Out"="074820", "error in"=w348) -> ("error out"=w347:errorcluster)  [unwired: 13 in]
          }
          frame True {
            n108 = call "WSVCAP SHL Host TL RFFE Write - Multiple DUTs - Common Data.vi"("Data Out"="074800", "error in"=w357, "Log (T)"=FALSE) -> ("error out"=w353:errorcluster)  [unwired: 12 in]
            n109 = case shown="2" "CP with DVA ON" {
              selector: "CP with DVA ON" -> [w363 w368 w373 w378 w382]
              tunnel: string[] ["07442F", "074436", "074428", "074429", "07443B"] -> [w364 w369 w374 w379 w384]
              tunnel: [w362 w367 w372 w377 w383] -> w349
              tunnel: ["35.0" ("Data Out") "29.75" ("Data Out") "30.5" ("Data Out") "44.0" ("Data Out") "40.25" ("Data Out")] -> _
              tunnel: w353 -> [w360 w365 w370 w375 w380]
              tunnel: [w360 w365 w370 w375 w380] -> w352
              frame 0, Default {
                n110 = Index Array(array=w364, index=w363) -> (element=w362:string)
              }
              frame 2 {
                n111 = Index Array(array=w369, index=w368) -> (element=w367:string)
              }
              frame 3 {
                n112 = Index Array(array=w374, index=w373) -> (element=w372:string)
              }
              frame 4 {
                n113 = Index Array(array=w379, index=w378) -> (element=w377:string)
              }
              frame 1 {
                n114 = Index Array(array=w384, index=w382) -> (element=w383:string)
              }
            }
            n115 = call "WSVCAP SHL Host TL RFFE Write - Multiple DUTs - Common Data.vi"("Data Out"=w349, "error in"=w352, "Log (T)"=FALSE) -> ("error out"=w355:errorcluster)  [unwired: 12 in]
          }
        }
        n116 = for {
          N: 36 -> [_]
          tunnel: "Serial Number" -> [w330]
          tunnel: [w328] -> w280 mode=indexing
          i -> [w327]
          n117 = Increment(x=w327) -> (x+1=w326:i32)
          n118 = Index Array(array=w330, index (row)=w326, index (col)=1 ("disabled index (col)")) -> (element=w328:string)
        }
        n119 = Not(x=w272) -> (.not. x?=w279:bool)
        n120 = Number To Fractional String(number="Set VDD", precision (6)=i16 2) -> (F-format string=w297:string)  [unwired: 2 in]
        n121 = call "Delay T4.vi"("milliseconds to wait"=w283, "error in (no error)"=w299) -> ("error out"=w287:errorcluster)  [unwired: 9 in]
        n122 = case shown="True" w276 {
          tunnel: w287 -> [w334 w336]
          tunnel: [w331 w335] -> w286
          tunnel: ["CAL OFF" ("Data Out") "CAL ON" ("Data Out")] -> w288
          frame False {
            n123 = call "WSVCAP SHL Host TL RFFE Write - Multiple DUTs - Common Data.vi"("Data Out"="074044", "error in"=w334) -> ("error out"=w331:errorcluster)  [unwired: 13 in]
          }
          frame True {
            n124 = for {
              tunnel: string[] ["074900", "074920", "074900"] -> [w344] mode=indexing
              tunnel: w336 -> [w341]
              tunnel: [w340] -> w335
              n125 = call "WSVCAP SHL Host TL RFFE Write - Multiple DUTs - Common Data.vi"("Data Out"=w344, "error in"=w341, "Log (T)"=FALSE) -> ("error out"=w343:errorcluster)  [unwired: 12 in]
              n126 = call "Delay T4.vi"("milliseconds to wait"=u32 10, "error in (no error)"=w343) -> ("error out"=w340:errorcluster)  [unwired: 9 in]
            }
          }
        }
        n127 = for {
          N: w306 -> [_]
          tunnel: w325 -> [w424]
          tunnel: [w420] -> w321
          tunnel: w294 -> [w419]
          tunnel: w314 -> [w418]
          tunnel: "TMN DC\\CAP Data Log File Path" -> [w417]
          tunnel: w312 -> [w415]
          tunnel: [w414] -> w310
          tunnel: w307 -> [w389]
          shift-right: [w409] -> _
          shift-left: u64 0 -> [w411]
          tunnel: w277 -> [w408]
          tunnel: w303 -> [w403]
          tunnel: w303 -> [w402]
          tunnel: w300 -> [w401]
          tunnel: w297 -> [w400]
          tunnel: [w399] -> w291
          tunnel: w288 -> [w398]
          tunnel: w286 -> [w397]
          tunnel: w275 -> [w396]
          tunnel: w278 -> [w394]
          tunnel: w274 -> [w393]
          tunnel: w279 -> [w392]
          tunnel: w273 -> [w391]
          tunnel: w280 -> [w390]
          tunnel: [w389] -> w269
          tunnel: w266 -> [w388]
          tunnel: w265 -> [w387]
          i -> [w407]
          stop <- w395 stop-if-true
          n128 = while {
            tunnel: w424 -> [w438]
            tunnel: w417 -> [w668]
            tunnel: "Lot#" -> [w667]
            tunnel: "Wafer#" -> [w666]
            tunnel: w390 -> [w665]
            tunnel: "Test Program" -> [w664]
            tunnel: w390 -> [w663]
            tunnel: "Comment" -> [w662]
            tunnel: "Lot#" -> [w661]
            tunnel: "Wafer#" -> [w660]
            tunnel: w418 -> [w657]
            tunnel: [w659] -> w420
            tunnel: w419 -> [w656]
            tunnel: w415 -> [w653]
            tunnel: [w652] -> w414
            tunnel: [w561] -> w405
            tunnel: w407 -> [w598]
            tunnel: [w589] -> w409
            tunnel: w411 -> [w588]
            shift-right: [w587] -> _
            shift-left: u64 0 -> [w488]
            tunnel: [w586] -> w404
            tunnel: w408 -> [w585]
            tunnel: w403 -> [w560]
            tunnel: w402 -> [w558]
            tunnel: w401 -> [w506]
            tunnel: w400 -> [w504]
            tunnel: [w485] -> w399
            tunnel: w398 -> [w491]
            tunnel: w397 -> [w439]
            tunnel: w396 -> [w490]
            tunnel: w394 -> [w482]
            tunnel: w393 -> [w481]
            tunnel: w392 -> [w476]
            tunnel: w391 -> [w470]
            tunnel: w388 -> [w446]
            tunnel: w387 -> [w445]
            i -> [w443]
            stop <- w599 stop-if-true
            n129 = Array Size(array=w438) -> (size(s)=w437:i32[])
            n130 = Index Array(array=w438, index (row)=w443, index (col)=0 ("disabled index (col)")) -> (element=w435:dbl)
            n131 = Index Array(array=w437, index=0) -> (element=w426:i32)
            n132 = call "CP_Cmd_Setting.vi"("error in (no error)"=w439, "Input"=w435) -> ("error out"=w442:errorcluster, "CP Voltage"=w440:string, "Send Cmd"=w441:string)  [unwired: 6 in, 1 out]
            "CP Voltage" <- w440
            n133 = To Unsigned Quad Integer(1:w426) -> (0:w425:u64)
            n134 = flat-sequence {
              tunnel: [w733] -> w651
              tunnel: [w730] -> w650
              tunnel: [w732] -> w649
              tunnel: w657 -> [w712]
              tunnel: w656 -> [w731]
              tunnel: [w731] -> w648
              tunnel: [w685] -> w647
              tunnel: [w682] -> w646
              tunnel: w442 -> [w725]
              tunnel: w598 -> [w728]
              tunnel: w443 -> [w708]
              tunnel: [w708] -> w595
              tunnel: w585 -> [w727]
              tunnel: [w726] -> w584
              tunnel: [w691] -> w579
              tunnel: [w690] -> w578
              tunnel: [w689] -> w577
              tunnel: [w695] -> w567
              tunnel: [w692] -> w566
              tunnel: w560 -> [w724]
              tunnel: [w724] -> w559
              tunnel: w558 -> [w723]
              tunnel: [w694] -> w545
              tunnel: [w693] -> w519
              tunnel: [w722] -> w507
              tunnel: w441 -> [w720]
              tunnel: [w709] -> w503
              tunnel: [w672] -> w495
              tunnel: w482 -> [w705]
              tunnel: w481 -> [w704]
              tunnel: [w704] -> w480
              tunnel: w476 -> [w703]
              tunnel: [w703] -> w475
              tunnel: w470 -> [w702]
              tunnel: [w702] -> w469
              tunnel: [w698] -> w464
              tunnel: ["Test Sequences"] -> w460
              tunnel: "Real No. From\nLookup Table" -> [w688]
              tunnel: ["WS1050/51"] -> w454
              tunnel: ["Cmin/Act"] -> w450
              tunnel: w446 -> [w677]
              tunnel: w445 -> [w676]
              tunnel: w435 -> [w675]
              tunnel: w425 -> [w669]
              tunnel: w435 -> [w670]
              tunnel: [w669] -> w434
              tunnel: w651 -> [w1024]
              tunnel: [w1020] -> w557
              tunnel: w650 -> [w1023]
              tunnel: w649 -> [w1029]
              tunnel: [w1029] -> w556
              tunnel: w648 -> [w1028]
              tunnel: w647 -> [w1022]
              tunnel: w646 -> [w1021]
              tunnel: [w1011] -> w555
              tunnel: [w1028] -> w554
              tunnel: [w1022] -> w553
              tunnel: [w1021] -> w552
              tunnel: w595 -> [w1026]
              tunnel: [w1026] -> w551
              tunnel: w584 -> [w1025]
              tunnel: [w1025] -> w550
              tunnel: [w1023] -> w549
              tunnel: w579 -> [w1019]
              tunnel: w578 -> [w1004]
              tunnel: w577 -> [w1005]
              tunnel: [w1016] -> w548
              tunnel: w567 -> [w1018]
              tunnel: w566 -> [w1016]
              tunnel: [w1012] -> w547
              tunnel: w559 -> [w1017]
              tunnel: [w1002] -> w546
              tunnel: w545 -> [w1002]
              tunnel: [w1004] -> w544
              tunnel: w519 -> [w1003]
              tunnel: [w1003] -> w518
              tunnel: [w1005] -> w516
              tunnel: w507 -> [w1015]
              tunnel: [w1014] -> w496
              tunnel: w495 -> [w1014]
              tunnel: w480 -> [w1010]
              tunnel: [w1010] -> w479
              tunnel: w475 -> [w1009]
              tunnel: [w1009] -> w474
              tunnel: w469 -> [w1008]
              tunnel: [w1008] -> w468
              tunnel: w464 -> [w1007]
              tunnel: [w1006] -> w463
              tunnel: w460 -> [w1000]
              tunnel: [w1000] -> w459
              tunnel: w454 -> [w999]
              tunnel: [w999] -> w453
              tunnel: w450 -> [w998]
              tunnel: [w998] -> w449
              tunnel: w434 -> [w997]
              tunnel: [w997] -> w433
              tunnel: w557 -> [w1144]
              tunnel: [w1143] -> w543
              tunnel: w556 -> [w1155]
              tunnel: [w1155] -> w540
              tunnel: w555 -> [w1135]
              tunnel: [w1135] -> w538
              tunnel: w554 -> [w1154]
              tunnel: [w1154] -> w536
              tunnel: w553 -> [w1153]
              tunnel: [w1153] -> w534
              tunnel: w552 -> [w1152]
              tunnel: [w1152] -> w532
              tunnel: w551 -> [w1151]
              tunnel: [w1151] -> w530
              tunnel: w550 -> [w1150]
              tunnel: [w1150] -> w528
              tunnel: w549 -> [w1149]
              tunnel: [w1149] -> w526
              tunnel: w548 -> [w1148]
              tunnel: [w1148] -> w524
              tunnel: [w1140] -> w522
              tunnel: w547 -> [w1139]
              tunnel: w546 -> [w1146]
              tunnel: w544 -> [w1145]
              tunnel: w518 -> [w1132]
              tunnel: [w1132] -> w517
              tunnel: w516 -> [w1134]
              tunnel: [w1134] -> w515
              tunnel: [w1141] -> w514
              tunnel: [w1142] -> w497
              tunnel: w496 -> [w1142]
              tunnel: w479 -> [w1138]
              tunnel: [w1138] -> w478
              tunnel: w474 -> [w1137]
              tunnel: [w1137] -> w473
              tunnel: w468 -> [w1136]
              tunnel: [w1136] -> w467
              tunnel: w463 -> [w1133]
              tunnel: w459 -> [w1130]
              tunnel: [w1133] -> w458
              tunnel: [w1130] -> w457
              tunnel: w453 -> [w1129]
              tunnel: [w1129] -> w452
              tunnel: w449 -> [w1128]
              tunnel: [w1128] -> w448
              tunnel: w433 -> [w1127]
              tunnel: [w1127] -> w432
              tunnel: w543 -> [w1237]
              tunnel: [w1236] -> w542
              tunnel: [w1232] -> w541
              tunnel: w540 -> [w1249]
              tunnel: [w1249] -> w539
              tunnel: w538 -> [w1226]
              tunnel: [w1226] -> w537
              tunnel: w536 -> [w1248]
              tunnel: [w1248] -> w535
              tunnel: w534 -> [w1247]
              tunnel: [w1247] -> w533
              tunnel: w532 -> [w1246]
              tunnel: [w1246] -> w531
              tunnel: w530 -> [w1245]
              tunnel: [w1245] -> w529
              tunnel: w528 -> [w1244]
              tunnel: [w1244] -> w527
              tunnel: w526 -> [w1243]
              tunnel: [w1243] -> w525
              tunnel: w524 -> [w1242]
              tunnel: [w1242] -> w523
              tunnel: w522 -> [w1241]
              tunnel: [w1241] -> w521
              tunnel: [w1223] -> w520
              tunnel: w517 -> [w1239]
              tunnel: w515 -> [w1238]
              tunnel: w514 -> [w1231]
              tunnel: ["DeltaC Target Setting(pF)"] -> w505
              tunnel: [w1234] -> w498
              tunnel: w497 -> [w1234]
              tunnel: w490 -> [w1233]
              tunnel: [w1233] -> w489
              tunnel: w478 -> [w1230]
              tunnel: [w1230] -> w477
              tunnel: w473 -> [w1229]
              tunnel: [w1229] -> w472
              tunnel: w467 -> [w1228]
              tunnel: [w1228] -> w466
              tunnel: w458 -> [w1227]
              tunnel: w457 -> [w1224]
              tunnel: [w1223] -> w455
              tunnel: w452 -> [w1222]
              tunnel: [w1222] -> w451
              tunnel: w448 -> [w1221]
              tunnel: [w1221] -> w447
              tunnel: w432 -> [w1220]
              tunnel: [w1220] -> w431
              tunnel: [w1368] -> w645
              tunnel: [w1334] -> w644
              tunnel: w542 -> [w1372]
              tunnel: w541 -> [w1348]
              tunnel: [w1357] -> w643
              tunnel: [w1348] -> w642
              tunnel: [w1371] -> w641
              tunnel: [w1370] -> w640
              tunnel: w539 -> [w1369]
              tunnel: [w1369] -> w639
              tunnel: w537 -> [w1357]
              tunnel: w535 -> [w1367]
              tunnel: [w1367] -> w638
              tunnel: w533 -> [w1363]
              tunnel: [w1363] -> w637
              tunnel: w531 -> [w1362]
              tunnel: [w1362] -> w636
              tunnel: w529 -> [w1358]
              tunnel: [w1358] -> w594
              tunnel: w527 -> [w1366]
              tunnel: [w1366] -> w583
              tunnel: w525 -> [w1365]
              tunnel: [w1364] -> w580
              tunnel: w523 -> [w1360]
              tunnel: w521 -> [w1356]
              tunnel: [w1361] -> w576
              tunnel: [w1359] -> w575
              tunnel: [w1356] -> w570
              tunnel: w520 -> [w1355]
              tunnel: [w1342] -> w565
              tunnel: [w1341] -> w564
              tunnel: [w1340] -> w563
              tunnel: w505 -> [w1354]
              tunnel: [w1339] -> w499
              tunnel: w498 -> [w1339]
              tunnel: [w1338] -> w494
              tunnel: w489 -> [w1337]
              tunnel: w477 -> [w1332]
              tunnel: w472 -> [w1331]
              tunnel: [w1331] -> w471
              tunnel: w466 -> [w1330]
              tunnel: [w1330] -> w465
              tunnel: w455 -> [w1327]
              tunnel: w451 -> [w1326]
              tunnel: w447 -> [w1315]
              tunnel: w431 -> [w1314]
              tunnel: [w1314] -> w430
              tunnel: w645 -> [w1576]
              tunnel: [w1576] -> w635
              tunnel: [w1561] -> w634
              tunnel: [w1575] -> w633
              tunnel: w644 -> [w1574]
              tunnel: w643 -> [w1573]
              tunnel: w642 -> [w1572]
              tunnel: [w1573] -> w632
              tunnel: [w1572] -> w631
              tunnel: w641 -> [w1571]
              tunnel: [w1571] -> w630
              tunnel: w640 -> [w1570]
              tunnel: [w1570] -> w629
              tunnel: w639 -> [w1569]
              tunnel: [w1569] -> w628
              tunnel: w638 -> [w1568]
              tunnel: [w1568] -> w627
              tunnel: w637 -> [w1567]
              tunnel: [w1567] -> w626
              tunnel: w636 -> [w1566]
              tunnel: [w1566] -> w625
              tunnel: w653 -> [w1565]
              tunnel: [w1563] -> w624
              tunnel: [w1543] -> w623
              tunnel: [w1544] -> w622
              tunnel: [w1542] -> w621
              tunnel: w594 -> [w1559]
              tunnel: [w1559] -> w593
              tunnel: w583 -> [w1558]
              tunnel: [w1558] -> w582
              tunnel: w580 -> [w1575]
              tunnel: w576 -> [w1556]
              tunnel: w575 -> [w1557]
              tunnel: [w1557] -> w574
              tunnel: [w1556] -> w572
              tunnel: w570 -> [w1555]
              tunnel: [w1555] -> w569
              tunnel: w565 -> [w1541]
              tunnel: w564 -> [w1540]
              tunnel: w563 -> [w1539]
              tunnel: [w1536] -> w562
              tunnel: [w1541] -> w513
              tunnel: [w1540] -> w511
              tunnel: [w1539] -> w509
              tunnel: [w1538] -> w500
              tunnel: w499 -> [w1538]
              tunnel: w494 -> [w1537]
              tunnel: [w1537] -> w493
              tunnel: w471 -> [w1536]
              tunnel: w465 -> [w1535]
              tunnel: w430 -> [w1534]
              tunnel: [w1534] -> w429
              tunnel: w635 -> [w1672]
              tunnel: [w1672] -> w620
              tunnel: w634 -> [w1696]
              tunnel: [w1695] -> w619
              tunnel: w668 -> [w1697]
              tunnel: w667 -> [w1694]
              tunnel: w666 -> [w1693]
              tunnel: w665 -> [w1692]
              tunnel: [w1691] -> w618
              tunnel: w633 -> [w1685]
              tunnel: [w1685] -> w617
              tunnel: w632 -> [w1690]
              tunnel: w631 -> [w1689]
              tunnel: [w1690] -> w616
              tunnel: [w1689] -> w615
              tunnel: [w1680] -> w614
              tunnel: w630 -> [w1688]
              tunnel: [w1688] -> w613
              tunnel: w629 -> [w1687]
              tunnel: [w1687] -> w612
              tunnel: w628 -> [w1684]
              tunnel: [w1686] -> w611
              tunnel: w488 -> [w1683]
              tunnel: [w1682] -> w610
              tunnel: [w1670] -> w609
              tunnel: w627 -> [w1681]
              tunnel: w626 -> [w1679]
              tunnel: w625 -> [w1678]
              tunnel: "File Name" -> [w1677]
              tunnel: w624 -> [w1676]
              tunnel: [w1676] -> w608
              tunnel: w623 -> [w1675]
              tunnel: [w1675] -> w607
              tunnel: [w1674] -> w606
              tunnel: w622 -> [w1674]
              tunnel: w621 -> [w1673]
              tunnel: [w1673] -> w605
              tunnel: [w1668] -> w596
              tunnel: w593 -> [w1669]
              tunnel: [w1669] -> w591
              tunnel: w588 -> [w1667]
              tunnel: w582 -> [w1666]
              tunnel: [w1666] -> w581
              tunnel: w574 -> [w1665]
              tunnel: [w1665] -> w573
              tunnel: w572 -> [w1664]
              tunnel: [w1664] -> w571
              tunnel: w569 -> [w1663]
              tunnel: [w1663] -> w568
              tunnel: w562 -> [w1662]
              tunnel: w513 -> [w1661]
              tunnel: [w1661] -> w512
              tunnel: w511 -> [w1660]
              tunnel: [w1660] -> w510
              tunnel: w509 -> [w1659]
              tunnel: [w1659] -> w508
              tunnel: w503 -> [w1658]
              tunnel: [w1658] -> w502
              tunnel: [w1657] -> w501
              tunnel: w500 -> [w1657]
              tunnel: w493 -> [w1656]
              tunnel: [w1656] -> w492
              tunnel: ["Freq(Hz)"] -> w462
              tunnel: ["Board#"] -> w461
              tunnel: w429 -> [w1653]
              tunnel: [w1653] -> w428
              tunnel: w620 -> [w1770]
              tunnel: w619 -> [w1769]
              tunnel: w668 -> [w1732]
              tunnel: w664 -> [w1764]
              tunnel: w663 -> [w1767]
              tunnel: w662 -> [w1763]
              tunnel: w661 -> [w1766]
              tunnel: w660 -> [w1762]
              tunnel: w618 -> [w1765]
              tunnel: [w1770] -> w601
              tunnel: [w1768] -> w602
              tunnel: w617 -> [w1760]
              tunnel: [w1760] -> w603
              tunnel: w616 -> [w1759]
              tunnel: w615 -> [w1744]
              tunnel: w614 -> [w1758]
              tunnel: w613 -> [w1757]
              tunnel: w612 -> [w1746]
              tunnel: [w1754] -> w604
              tunnel: w611 -> [w1756]
              tunnel: w610 -> [w1755]
              tunnel: w609 -> [w1754]
              tunnel: "File Name" -> [w1725]
              tunnel: w608 -> [w1753]
              tunnel: [w1753] -> w600
              tunnel: w607 -> [w1752]
              tunnel: w606 -> [w1751]
              tunnel: w605 -> [w1750]
              tunnel: [w1749] -> w597
              tunnel: w596 -> [w1749]
              tunnel: [w1728] -> w592
              tunnel: w591 -> [w1728]
              tunnel: w581 -> [w1748]
              tunnel: w573 -> [w1747]
              tunnel: w571 -> [w1745]
              tunnel: w568 -> [w1743]
              tunnel: w512 -> [w1742]
              tunnel: w510 -> [w1741]
              tunnel: w508 -> [w1740]
              tunnel: w506 -> [w1739]
              tunnel: w491 -> [w1738]
              tunnel: w440 -> [w1737]
              tunnel: w504 -> [w1736]
              tunnel: w502 -> [w1735]
              tunnel: w501 -> [w1734]
              tunnel: w492 -> [w1733]
              tunnel: [w1730] -> w487
              tunnel: [w1721] -> w483
              tunnel: w462 -> [w1720]
              tunnel: w461 -> [w1718]
              tunnel: w428 -> [w1717]
              tunnel: [w1717] -> w427
              tunnel: [w1791] -> w658
              tunnel: [w1792] -> w659
              tunnel: [w1793] -> w561
              tunnel: w604 -> [w1784]
              tunnel: w603 -> [w1792]
              tunnel: w602 -> [w1781]
              tunnel: w601 -> [w1793]
              tunnel: w600 -> [w1786]
              tunnel: [w1786] -> w652
              tunnel: [w1783] -> w589
              tunnel: w597 -> [w1783]
              tunnel: w592 -> [w1785]
              tunnel: [w1785] -> w590
              tunnel: [w1784] -> w587
              tunnel: [w1782] -> w586
              tunnel: [w1780] -> w484
              tunnel: w487 -> [w1779]
              tunnel: w483 -> [w1777]
              tunnel: w427 -> [w1776]
              frame #0 {
                w699 = FALSE ("Log (T)")
                n135 = call "WSVCAP SHL Host TL RFFE Write - Multiple DUTs - Common Data.vi"("Data Out"=w720, "error in"=w725, "Log (T)"=FALSE) -> ("error out"=w706:errorcluster)  [unwired: 12 in]
                n136 = for {
                  tunnel: string[] ["0760", "0767", "0768"] -> [w755] mode=indexing
                  tunnel: [w751] -> w710 mode=indexing
                  tunnel: w706 -> [w749]
                  tunnel: [w748] -> w707
                  i -> [w754]
                  n137 = call "Delay T4.vi"("milliseconds to wait"=u32 10, "error in (no error)"=w749) -> ("error out"=w756:errorcluster)  [unwired: 9 in]
                  n138 = call "WSVCAP SHL Host TL RFFE Read - Multiple DUTs - Common Data.vi"("Data Out"=w755, "error in"=w756, "Log (T)"=FALSE) -> ("RFFE Data In"=w753:string[], "error out"=w748:errorcluster)  [unwired: 11 in]
                  n139 = Index Array(array=w753, index=w754) -> (element=w750:string)
                  n140 = String Subset(string=w750, offset (0)=0) -> (substring=w751:string)  [unwired: 1 in]
                }
                "RB Reg for HD/Cycle" <- w710
                n141 = local read "IDD Brd(uA)"() -> (w719:string)
                n142 = call "Delay T4.vi"("milliseconds to wait"=u32 100, "error in (no error)"=w707) -> ("error out"=w715:errorcluster)  [unwired: 9 in]
                n143 = call "Ke2000 Single Reading.vi"("error in (no error)"=w715, "VISA resource name"=w712) -> ("error out"=w717:errorcluster, "VISA resource name out"=w687:refnum<visa-resource-name>, "uA"=w718:string)  [unwired: 5 in, 2 out]
                n144 = call "Substration.vi"("error in (no error)"=w717, "Input2"=w719, "Input1"=w718) -> ("error out"=w714:errorcluster, "In1 - In2"=→"IDD_HD/CYC (uA)":string)  [unwired: 7 in]
                n145 = case shown="True" w727 {
                  tunnel: [w787 w892] -> w733
                  tunnel: [w788 w877] -> w671
                  tunnel: [w786 w893] -> w732
                  tunnel: w714 -> [w782 w881]
                  tunnel: w728 -> [_ w883]
                  tunnel: w675 -> [w779 w878]
                  tunnel: [w784 w879] -> w726
                  tunnel: w708 -> [w771 w875]
                  tunnel: w723 -> [w781 _]
                  tunnel: ["% Duty Cycle" "100" ("Data Out")] -> w709
                  tunnel: w705 -> [w769 _]
                  tunnel: w688 -> [w768 w870]
                  tunnel: w677 -> [w765 _]
                  tunnel: w676 -> [w764 _]
                  frame False {
                    # "Cycles in 1s"
                    n146 = case shown="True" w768 {
                      tunnel: w782 -> [w794 w800]
                      tunnel: w779 -> [w793 w799]
                      tunnel: [w792 w800] -> w778
                      tunnel: w771 -> [w791 _]
                      tunnel: [w790 w799] -> w777
                      tunnel: [u64 1000 ("y") u64 1 ("y")] -> w772
                      frame False {
                        n147 = case shown="8, Default" w791 {
                          tunnel: w793 -> [w796 _]
                          tunnel: [w796 "Cycle RP"] -> w790
                          tunnel: [w795 w797] -> w792
                          tunnel: w794 -> [w795 w797]
                          frame 0..7 {
                          }
                          frame 8, Default {
                          }
                        }
                      }
                      frame True {
                        # "Read real number\nfrom lookup table"
                      }
                    }
                    n148 = call "WSVCAP SHL Host TL RFFE Configure.vi"("RFFE Slave Address"=w781, "Clock Rate (Hz)"="SPI Clock Rate (Hz)", "error in"=w778) -> ("Actual Rate (Hz)"=→"AR Cycling(Hz)":dbl, "error out"=w767:errorcluster)  [unwired: 11 in]
                    n149 = Array Max & Min(array=w764) -> (max value=w775:dbl)  [unwired: 3 out]
                    n150 = Divide(x=1.0, y=w775) -> (x/y=w774:dbl)
                    n151 = To Unsigned Quad Integer(1:w774) -> (0:w773:u64)
                    n152 = Not(x=w769) -> (.not. x?=w770:bool)
                    n153 = case shown="False" w770 {
                      tunnel: [w803 w825] -> w788
                      tunnel: [w806 w824] -> w787
                      tunnel: [u64 1 w823] -> w786
                      tunnel: w767 -> [w804 w822]
                      tunnel: w777 -> [_ w821]
                      tunnel: w764 -> [_ w819]
                      tunnel: w773 -> [_ w818]
                      tunnel: w772 -> [_ w817]
                      tunnel: w771 -> [w802 _]
                      tunnel: w765 -> [_ w816]
                      frame False {
                        n154 = case shown="1, Default" w802 {
                          tunnel: w804 -> [w807 w809]
                          tunnel: [w807 w808] -> w803
                          frame 0 {
                          }
                          frame 1, Default {
                            n155 = flat-sequence {
                              tunnel: "Repeat Meas(s)" -> [w815]
                              tunnel: w809 -> [w812]
                              tunnel: [w812] -> w808
                              frame #0 {
                                n156 = Multiply(x=w815, y=u32 1000) -> (x*y=w814:u32)
                                n157 = Wait (ms)(milliseconds to wait=w814) -> ()  [unwired: 1 out]
                                n158 = local write "STATUS"("Verify Sockets waiting times..." ("STATUS")) -> ()
                              }
                            }
                          }
                        }
                        n159 = local read "stop During HD/Cycles"() -> (w806:bool)
                      }
                      frame True {
                        n160 = while {
                          tunnel: w821 -> [w845]
                          tunnel: [w832] -> w825
                          tunnel: [w837] -> w824
                          tunnel: w822 -> [w843]
                          tunnel: [w831] -> w823
                          tunnel: w816 -> [w842]
                          tunnel: w819 -> [w841]
                          tunnel: w818 -> [w828]
                          tunnel: w817 -> [w826]
                          i -> [w840]
                          stop <- w836 stop-if-true
                          # "At least 1 second before target"
                          # "Remaining Cycles"
                          # "Target Cycles"
                          # "Cycles in 1s"
                          n161 = To Unsigned Quad Integer(1:w845) -> (0:w844:u64)
                          n162 = case shown="0" w840 {
                            tunnel: [w853 w855] -> w834
                            tunnel: w843 -> [w854 w855]
                            tunnel: w842 -> [w852 _]
                            tunnel: w841 -> [w851 _]
                            frame 0 {
                              n163 = call "WSVCAP SHL Host TL RFFE Write Cycle - Multiple DUTs - Common Data.vi"("Data Out (Cycle Commands)"=w852, "Post Command Delay"=w851, "error in"=w854, "Log (T)"=FALSE) -> ("error out"=w853:errorcluster)  [unwired: 11 in]
                            }
                            frame 1, Default {
                            }
                          }
                          n164 = Multiply(x=w844, y=w826) -> (x*y=w831:u64)
                          n165 = call "WSVCAP SHL Host TL SPI_RFFE Query Cycle Count.vi"("error in"=w834) -> ("Cycle Count"=w830:u64, "error out"=w839:errorcluster)  [unwired: 13 in]
                          "Cycle Count" <- w830
                          n166 = Subtract(x=w831, y=w830) -> (x-y=w829:u64)
                          n167 = Greater Or Equal?(x=w830, y=w831) -> (x >= y?=w838:bool)
                          n168 = local read "stop During HD/Cycles"() -> (w837:bool)
                          n169 = Greater?(x=w829, y=w828) -> (0:w827:bool)
                          n170 = case shown="True" w838 {
                            tunnel: [w857 w860] -> w833
                            tunnel: w839 -> [w857 w859]
                            tunnel: [FALSE TRUE] -> w835
                            frame False {
                            }
                            frame True {
                              n171 = call "WSVCAP SHL Host TL SPI Stop Write Cycle.vi"("error in"=w859) -> ("error out"=w860:errorcluster)  [unwired: 14 in]
                            }
                          }
                          n172 = Or(x=w835, y=w837) -> (x .or. y?=w836:bool)
                          n173 = case shown="True" w827 {
                            tunnel: w833 -> [w846 w849]
                            tunnel: [w846 w848] -> w832
                            frame False {
                            }
                            frame True {
                              n174 = call "MISC Wait with Data Flow.vi"("Error In (no error)"=w849, "Wait Time (500ms)"=u32 50) -> ("Error Out"=w848:errorcluster)  [unwired: 7 in, 2 out]
                            }
                          }
                        }
                        n175 = local write "STATUS"("Parts are Cycling...." ("STATUS")) -> ()
                      }
                    }
                    n176 = local read "HD/CYC Temp"() -> (w783:i32)
                    n177 = Number To Engineering String(4:w783) -> (0:w784:string)  [unwired: 3 in]
                  }
                  frame True {
                    n178 = case shown="False" w870 {
                      tunnel: w883 -> [w910 _]
                      tunnel: [w909 w922] -> w882
                      tunnel: w881 -> [w908 w923]
                      tunnel: [w907 w923] -> w880
                      tunnel: w878 -> [w906 w922]
                      tunnel: w875 -> [w905 _]
                      frame False {
                        n179 = case shown="1, Default" w910 {
                          tunnel: [w913 w920] -> w909
                          tunnel: w908 -> [w915 w921]
                          tunnel: [w914 w921] -> w907
                          tunnel: w906 -> [w912 _]
                          tunnel: w905 -> [w911 _]
                          frame 0 {
                            n180 = case shown="15, Default" w911 {
                              tunnel: [w916 "HD RP"] -> w913
                              tunnel: w915 -> [w917 w918]
                              tunnel: [w917 w918] -> w914
                              tunnel: w912 -> [w916 _]
                              frame 0..14 {
                              }
                              frame 15, Default {
                              }
                            }
                          }
                          frame 1, Default {
                            n181 = local read "HD RP"() -> (w920:dbl)
                          }
                        }
                      }
                      frame True {
                      }
                    }
                    n182 = call "WSVCAP SHL Host TL RFFE Write - Multiple DUTs - Common Data.vi"("Data Out"="Cmd To HD", "error in"=w880, "Log (T)"=FALSE) -> ("error out"=w866:errorcluster)  [unwired: 12 in]
                    n183 = local read "No of HD/Cycle\nCompleted"() -> (w884:u64)
                    n184 = call "Delay T4.vi"("milliseconds to wait"=u32 50, "error in (no error)"=w866) -> ("error out"=w863:errorcluster)  [unwired: 9 in]
                    n185 = for {
                      tunnel: string[] ["0761", "0762", "0763"] -> [w904] mode=indexing
                      tunnel: [w900] -> w862 mode=indexing
                      shift-right: [w897] -> w888
                      shift-left: w863 -> [w903]
                      i -> [w902]
                      n186 = call "WSVCAP SHL Host TL RFFE Read - Multiple DUTs - Common Data.vi"("Data Out"=w904, "error in"=w903, "Log (T)"=FALSE) -> ("RFFE Data In"=w899:string[], "error out"=w896:errorcluster)  [unwired: 11 in]
                      n187 = Index Array(array=w899, index=w902) -> (element=w898:string)
                      n188 = call "Delay T4.vi"("milliseconds to wait"=u32 10, "error in (no error)"=w896) -> ("error out"=w897:errorcluster)  [unwired: 9 in]
                      n189 = String Subset(string=w898, offset (0)=0) -> (substring=w900:string)  [unwired: 1 in]
                    }
                    "RB Reg for HD" <- w862
                    n190 = Greater?(x="HD_DC (Min)", y=w884) -> (0:w885:bool)
                    n191 = case shown="True" w885 {
                      tunnel: [_ w934] -> w890
                      tunnel: [w925 w933] -> w889
                      tunnel: w888 -> [w925 w932]
                      tunnel: w882 -> [w924 w931]
                      tunnel: [w924 w931] -> w887
                      frame False {
                      }
                      frame True {
                        n192 = Multiply(x=1000.0, y=w931) -> (x*y=w929:dbl)
                        n193 = Multiply(x=60.0, y=w929) -> (x*y=w927:dbl)
                        n194 = local write "STATUS"("Parts are Holding Down..." ("STATUS")) -> ()
                        n195 = event shown="[0] Timeout" {
                          selector: _ -> [_ _]
                          dyn-events: _ -> [_ _]
                          timeout: w927 -> [_ _]
                          tunnel: ["stop During HD/Cycles" TRUE ("stop During HD/Cycles")] -> w934
                          tunnel: w932 -> [w935 w937]
                          tunnel: [w935 w937] -> w933
                          event Timeout {
                            n196 = event-data() -> ()  [unwired: 1 in, 2 out]
                          }
                          event "stop During HD/Cycles": Value Change {
                            n197 = event-data() -> ()  [unwired: 1 in, 2 out]
                          }
                        }
                      }
                    }
                    n198 = Greater Or Equal?(x=w884, y="HD_DC (Min)") -> (x >= y?=w891:bool)
                    n199 = To Unsigned Quad Integer(1:w882) -> (0:w893:u64)
                    n200 = Add(x="Time All OFF (s)", y="Time All ON (s)") -> (x+y=w872:u32)
                    n201 = To Double Precision Float(number=w872) -> (double precision float=w871:dbl)
                    n202 = Divide(x=w871, y=60.0) -> (x/y=w873:dbl)
                    n203 = case shown="True" w891 {
                      tunnel: [w941 w957] -> w892
                      tunnel: [w942 w949] -> w877
                      tunnel: w889 -> [w942 w956]
                      tunnel: w890 -> [w941 w955]
                      tunnel: w887 -> [_ w954]
                      tunnel: [w940 w952] -> w879
                      tunnel: w873 -> [_ w946]
                      tunnel: "Time All OFF (s)" -> [_ w944]
                      tunnel: "Time All ON (s)" -> [_ w943]
                      frame False {
                        n204 = Number To Engineering String(4:"HD/CYC Temp") -> (0:w940:string)  [unwired: 3 in]
                      }
                      frame True {
                        n205 = Divide(x=w954, y=w946) -> (x/y=w953:dbl)
                        n206 = call "WSVCAP SHL Host TL RFFE Write - Multiple DUTs - Common Data.vi"("Data Out"="070201000000", "error in"=w956, "Log (T)"=FALSE) -> ("error out"=w959:errorcluster)  [unwired: 12 in]
                        n207 = Round To Nearest(number=w953) -> (nearest integer value=w948:dbl)
                        n208 = call "Delay T4.vi"("milliseconds to wait"=u32 50, "error in (no error)"=w959) -> ("error out"=w950:errorcluster)  [unwired: 9 in]
                        n209 = To Long Integer(number=w948) -> (32bit integer=w947:i32)
                        "No LPs to RP" <- w947
                        n210 = for {
                          N: w947 -> [_]
                          tunnel: w955 -> [w977]
                          tunnel: [w976] -> w957
                          tunnel: w950 -> [w966]
                          tunnel: [w965] -> w949
                          tunnel: w944 -> [w963]
                          tunnel: w943 -> [w961]
                          i -> [w975]
                          stop <- w976 stop-if-true
                          w964 = FALSE ("Log (T)")
                          w962 = u32 1 ("milliseconds to wait")
                          n211 = Increment(x=w975) -> (x+1=→"LPs Count":i32)
                          n212 = call "WSVCAP SHL Host TL RFFE Write - Multiple DUTs - Common Data.vi"("Data Out"="074776", "error in"=w966, "Log (T)"=w964) -> ("error out"=w983:errorcluster)  [unwired: 12 in]
                          n213 = call "Delay T4.vi"("milliseconds to wait"=w962, "error in (no error)"=w983) -> ("error out"=w982:errorcluster)  [unwired: 9 in]
                          n214 = local read "Set CP to Meas"() -> (w968:i32)
                          n215 = call "WSVCAP SHL Host TL RFFE Write - Multiple DUTs - Common Data.vi"("Data Out"="070201000000", "error in"=w969) -> ("error out"=w979:errorcluster)  [unwired: 13 in]
                          n216 = call "WSVCAP SHL Host TL RFFE Write - Multiple DUTs - Common Data.vi"("Data Out"="0702013B3B3B", "error in"=w982, "Log (T)"=w964) -> ("error out"=w972:errorcluster)  [unwired: 12 in]
                          n217 = call "Delay T4.vi"("milliseconds to wait"=w962, "error in (no error)"=w972) -> ("error out"=w971:errorcluster)  [unwired: 9 in]
                          n218 = flat-sequence {
                            tunnel: w979 -> [w990]
                            tunnel: [w988] -> w965
                            tunnel: w963 -> [w985]
                            frame #0 {
                              n219 = local write "STATUS"("Now HD OFF Time..." ("STATUS")) -> ()
                              n220 = Multiply(x=w985, y=u32 1000) -> (x*y=w987:u32)
                              n221 = call "Delay T4.vi"("milliseconds to wait"=w987, "error in (no error)"=w990) -> ("error out"=w988:errorcluster)  [unwired: 9 in]
                            }
                          }
                          n222 = Index Array(array=string[] ["07476F", "074776", "074765", "074769", "07477B"], index=w968) -> (element=w973:string)
                          n223 = call "WSVCAP SHL Host TL RFFE Write - Multiple DUTs - Common Data.vi"("Data Out"=w973, "error in"=w971, "Log (T)"=w964) -> ("error out"=w970:errorcluster)  [unwired: 12 in]
                          n224 = flat-sequence {
                            tunnel: [w995] -> w969
                            tunnel: w970 -> [w992]
                            tunnel: w961 -> [w991]
                            frame #0 {
                              n225 = local write "STATUS"("Now HD ON Time..." ("STATUS")) -> ()
                              n226 = Multiply(x=w991, y=u32 1000) -> (x*y=w994:u32)
                              n227 = call "Delay T4.vi"("milliseconds to wait"=w994, "error in (no error)"=w992) -> ("error out"=w995:errorcluster)  [unwired: 9 in]
                            }
                          }
                          n228 = Unbundle By Name(w965) -> ("status"=w978:bool)
                          n229 = Or(x=w978, y=w977) -> (x .or. y?=w976:bool)
                        }
                        n230 = Number To Engineering String(4:"DC_Temp") -> (0:w952:string)  [unwired: 3 in]
                      }
                    }
                  }
                }
                n231 = call "CP_Cmd_Setting.vi"("error in (no error)"=w671, "Input"=w670) -> ("error out"=w674:errorcluster, "CP Voltage"=w672:string, "Send Cmd"=w673:string)  [unwired: 6 in, 1 out]
                n232 = flat-sequence {
                  tunnel: w701 -> [w758]
                  tunnel: [w758] -> w697
                  frame #0 {
                    w760 = "0" ("NOM IDD OFF(uA)")
                    w761 = string[] []
                    w762 = string[][] []
                    n233 = local write "Total Delta C1(pF)"(w761) -> ()
                    n234 = local write "Total Delta C2(pF)"(w761) -> ()
                    n235 = local write "Total Delta C3(pF)"(w761) -> ()
                    n236 = local write "Current EFuse Read back"(w761) -> ()
                    n237 = local write "RB Reg for HD"(w761) -> ()
                    n238 = To Long Integer(number=0.0 ("No of Loops to RP")) -> (32bit integer=w759:i32)
                    n239 = local write "NOM IDD ON (uA)"(w760) -> ()
                    n240 = local write "NOM IDD OFF(uA)"(w760) -> ()
                    n241 = local write "LPs Count"(w759) -> ()
                    n242 = local write "No LPs to RP"(w759) -> ()
                    n243 = local write "VSA_V3"(w762) -> ()
                    n244 = local write "VSA_V1"(w762) -> ()
                    n245 = local write "VSA_V2"(w762) -> ()
                    n246 = local write "VPI C1"(w762) -> ()
                    n247 = local write "VPI C2"(w762) -> ()
                    n248 = local write "VPI C3"(w762) -> ()
                    n249 = local write "% Delta C"(w762) -> ()
                    n250 = local write "40V_3"(w762) -> ()
                    n251 = local write "40V_2"(w762) -> ()
                    n252 = local write "40V_1"(w762) -> ()
                  }
                }
                n253 = call "WSVCAP SHL Host TL RFFE Write - Multiple DUTs - Common Data.vi"("Data Out"=w673, "error in"=w674, "Log (T)"=w699) -> ("error out"=w721:errorcluster)  [unwired: 12 in]
                n254 = call "Delay T4.vi"("milliseconds to wait"=u32 50, "error in (no error)"=w721) -> ("error out"=w680:errorcluster)  [unwired: 9 in]
                n255 = for {
                  tunnel: [w746] -> w730
                  tunnel: [w745] -> w701
                  tunnel: w699 -> [w744]
                  tunnel: w687 -> [w743]
                  tunnel: w680 -> [w739]
                  tunnel: string[] ["0702013B3B3B", "070201000000"] -> [w735] mode=indexing
                  tunnel: [w734] -> w683 mode=indexing
                  n256 = call "WSVCAP SHL Host TL RFFE Write - Multiple DUTs - Common Data.vi"("Data Out"=w735, "error in"=w739, "Log (T)"=w744) -> ("error out"=w740:errorcluster)  [unwired: 12 in]
                  n257 = local read "IDD Brd(uA)"() -> (w736:string)
                  n258 = call "Delay T4.vi"("milliseconds to wait"=u32 100, "error in (no error)"=w740) -> ("error out"=w741:errorcluster)  [unwired: 9 in]
                  n259 = call "Ke2000 Single Reading.vi"("error in (no error)"=w741, "VISA resource name"=w743) -> ("error out"=w738:errorcluster, "VISA resource name out"=w746:refnum<visa-resource-name>, "uA"=w737:string)  [unwired: 5 in, 2 out]
                  n260 = call "Substration.vi"("error in (no error)"=w738, "Input2"=w736, "Input1"=w737) -> ("error out"=w745:errorcluster, "In1 - In2"=w734:string)  [unwired: 7 in]
                }
                n261 = Index Array(array=w683, index=1) -> (element=w682:string)
                n262 = Index Array(array=w683, index=0) -> (element=w685:string)
                n263 = local read "Clock Rate (Hz)"() -> (w722:dbl)
                n264 = call "Multi Dut Cmd_Header Setting.vi"("WS1050/51"="WS1050/51", "Cmin/Act"="Cmin/Act", "Test Seq"="Test Sequences", "error in (no error)"=w697) -> ("Name 1"=w695:string[], "Name 2"=w694:string[], "Name Header"=w692:string[], "Name 3"=w693:string[], "Cmd 3"=w689:string[], "Cmd 1"=w691:string[], "Cmd 2"=w690:string[], "error out"=w698:errorcluster)  [unwired: 2 in, 2 out]
                "Loops Run" <- w669
              }
              frame #1 {
                w1006 = FALSE ("Log (T)")
                n265 = call "WSVCAP SHL Host TL RFFE Configure.vi"("RFFE Slave Address"=w1017, "Clock Rate (Hz)"=w1015, "error in"=w1007) -> ("Actual Rate (Hz)"=w1027:dbl, "error out"=w1013:errorcluster)  [unwired: 11 in]
                n266 = local write "AR  Measurent(Hz)"(w1027) -> ()
                n267 = Array Size(array=w1018) -> (size(s)=w1030:i32)
                n268 = case shown="2" w1000 {
                  tunnel: w1030 -> [w1039 w1071 w1103]
                  tunnel: w1024 -> [w1038 w1070 w1102]
                  tunnel: [w1037 w1069 w1101] -> w1020
                  tunnel: w1019 -> [w1036 w1068 w1100]
                  tunnel: w1018 -> [w1035 w1067 w1099]
                  tunnel: w1013 -> [w1034 w1066 w1098]
                  tunnel: [w1033 w1065 w1097] -> w1012
                  tunnel: w1006 -> [w1032 w1064 w1096]
                  tunnel: [w1031 w1063 w1095] -> w1001
                  frame 0, Default {
                    n269 = for {
                      N: w1039 -> [_]
                      tunnel: w1036 -> [w1058]
                      tunnel: w1038 -> [w1056]
                      tunnel: [w1055] -> w1037
                      tunnel: [w1051] -> w1031 mode=indexing
                      tunnel: w1035 -> [w1053]
                      tunnel: w1034 -> [w1041]
                      tunnel: [w1043] -> w1033
                      tunnel: w1032 -> [w1042]
                      i -> [w1050]
                      stop <- w1055 stop-if-true
                      n270 = Index Array(array=w1058, index=w1050) -> (element=w1054:string)
                      n271 = Index Array(array=w1053, index=w1050) -> (element=w1052:string)
                      n272 = local write "STATUS"(w1052) -> ()
                      n273 = call "WSVCAP SHL Host TL RFFE Write - Multiple DUTs - Common Data.vi"("Data Out"=w1054, "error in"=w1041, "Log (T)"=FALSE) -> ("error out"=w1045:errorcluster)  [unwired: 12 in]
                      n274 = call "Delay T4.vi"("milliseconds to wait"=u32 10, "error in (no error)"=w1045) -> ("error out"=w1049:errorcluster)  [unwired: 9 in]
                      n275 = call "WS1050 AD7747 READ 36 DUT.vi"("error in"=w1049, "Log (T)"=w1042, "DUT Mask Mode (All)"=WSVCAP_SHL_I2C_DUT_Mask_Mode_Enum."C1") -> ("error out"=w1047:errorcluster, "AD7747 Values"=w1048:string[][])  [unwired: 7 in]
                      n276 = for {
                        tunnel: w1048 -> [w1061] mode=indexing
                        tunnel: w1047 -> [w1062]
                        tunnel: [w1062] -> w1043
                        tunnel: [w1059] -> w1051 mode=indexing
                        n277 = Index Array(array=w1061, index=1) -> (element=w1059:string)
                      }
                      n278 = Unbundle By Name(w1043) -> ("status"=w1057:bool)
                      n279 = Or(x=w1057, y=w1056) -> (x .or. y?=w1055:bool)
                    }
                  }
                  frame 1 {
                    n280 = for {
                      N: w1071 -> [_]
                      tunnel: w1068 -> [w1090]
                      tunnel: w1070 -> [w1088]
                      tunnel: [w1087] -> w1069
                      tunnel: [w1083] -> w1063 mode=indexing
                      tunnel: w1067 -> [w1085]
                      tunnel: w1066 -> [w1073]
                      tunnel: [w1075] -> w1065
                      tunnel: w1064 -> [w1074]
                      i -> [w1082]
                      stop <- w1087 stop-if-true
                      n281 = Index Array(array=w1090, index=w1082) -> (element=w1086:string)
                      n282 = Index Array(array=w1085, index=w1082) -> (element=w1084:string)
                      n283 = local write "STATUS"(w1084) -> ()
                      n284 = call "WSVCAP SHL Host TL RFFE Write - Multiple DUTs - Common Data.vi"("Data Out"=w1086, "error in"=w1073, "Log (T)"=FALSE) -> ("error out"=w1077:errorcluster)  [unwired: 12 in]
                      n285 = call "Delay T4.vi"("milliseconds to wait"=u32 10, "error in (no error)"=w1077) -> ("error out"=w1081:errorcluster)  [unwired: 9 in]
                      n286 = call "WS1050 AD7747 READ 36 DUT.vi"("error in"=w1081, "Log (T)"=w1074, "DUT Mask Mode (All)"=WSVCAP_SHL_I2C_DUT_Mask_Mode_Enum."C2") -> ("error out"=w1079:errorcluster, "AD7747 Values"=w1080:string[][])  [unwired: 7 in]
                      n287 = for {
                        tunnel: w1080 -> [w1093] mode=indexing
                        tunnel: w1079 -> [w1094]
                        tunnel: [w1094] -> w1075
                        tunnel: [w1091] -> w1083 mode=indexing
                        n288 = Index Array(array=w1093, index=3) -> (element=w1091:string)
                      }
                      n289 = Unbundle By Name(w1075) -> ("status"=w1089:bool)
                      n290 = Or(x=w1089, y=w1088) -> (x .or. y?=w1087:bool)
                    }
                  }
                  frame 2 {
                    n291 = for {
                      N: w1103 -> [_]
                      tunnel: w1100 -> [w1122]
                      tunnel: w1102 -> [w1120]
                      tunnel: [w1119] -> w1101
                      tunnel: [w1115] -> w1095 mode=indexing
                      tunnel: w1099 -> [w1117]
                      tunnel: w1098 -> [w1105]
                      tunnel: [w1107] -> w1097
                      tunnel: w1096 -> [w1106]
                      i -> [w1114]
                      stop <- w1119 stop-if-true
                      n292 = Index Array(array=w1122, index=w1114) -> (element=w1118:string)
                      n293 = Index Array(array=w1117, index=w1114) -> (element=w1116:string)
                      n294 = local write "STATUS"(w1116) -> ()
                      n295 = call "WSVCAP SHL Host TL RFFE Write - Multiple DUTs - Common Data.vi"("Data Out"=w1118, "error in"=w1105, "Log (T)"=FALSE) -> ("error out"=w1109:errorcluster)  [unwired: 12 in]
                      n296 = call "Delay T4.vi"("milliseconds to wait"=u32 10, "error in (no error)"=w1109) -> ("error out"=w1113:errorcluster)  [unwired: 9 in]
                      n297 = call "WS1050 AD7747 READ 36 DUT.vi"("error in"=w1113, "Log (T)"=w1106, "DUT Mask Mode (All)"=WSVCAP_SHL_I2C_DUT_Mask_Mode_Enum."C3") -> ("error out"=w1111:errorcluster, "AD7747 Values"=w1112:string[][])  [unwired: 7 in]
                      n298 = for {
                        tunnel: w1112 -> [w1125] mode=indexing
                        tunnel: w1111 -> [w1126]
                        tunnel: [w1126] -> w1107
                        tunnel: [w1123] -> w1115 mode=indexing
                        n299 = Index Array(array=w1125, index=5) -> (element=w1123:string)
                      }
                      n300 = Unbundle By Name(w1107) -> ("status"=w1121:bool)
                      n301 = Or(x=w1121, y=w1120) -> (x .or. y?=w1119:bool)
                    }
                  }
                }
                n302 = Transpose 2D Array(2D array=w1001) -> (transposed array=w1011:string[][])
                "40V_1" <- w1011
                "NOM IDD ON (uA)" <- w1022
                "NOM IDD OFF(uA)" <- w1021
              }
              frame #2 {
                n303 = Array Size(array=w1146) -> (size(s)=w1147:i32)
                n304 = case shown="0, 2, Default" w1130 {
                  tunnel: w1147 -> [w1164 w1196]
                  tunnel: w1146 -> [w1163 w1195]
                  tunnel: w1145 -> [w1162 w1194]
                  tunnel: w1144 -> [w1161 w1193]
                  tunnel: [w1160 w1192] -> w1143
                  tunnel: [w1159 w1191] -> w1141
                  tunnel: w1139 -> [w1158 w1190]
                  tunnel: w1133 -> [w1157 w1189]
                  tunnel: [w1156 w1188] -> w1131
                  frame 0, 2, Default {
                    n305 = for {
                      N: w1164 -> [_]
                      tunnel: w1162 -> [w1183]
                      tunnel: w1161 -> [w1181]
                      tunnel: [w1180] -> w1160
                      tunnel: [w1176] -> w1156 mode=indexing
                      tunnel: w1163 -> [w1178]
                      tunnel: w1158 -> [w1166]
                      tunnel: [w1168] -> w1159
                      tunnel: w1157 -> [w1167]
                      i -> [w1175]
                      stop <- w1180 stop-if-true
                      n306 = Index Array(array=w1183, index=w1175) -> (element=w1179:string)
                      n307 = Index Array(array=w1178, index=w1175) -> (element=w1177:string)
                      n308 = call "WSVCAP SHL Host TL RFFE Write - Multiple DUTs - Common Data.vi"("Data Out"=w1179, "error in"=w1166, "Log (T)"=FALSE) -> ("error out"=w1170:errorcluster)  [unwired: 12 in]
                      n309 = local write "STATUS"(w1177) -> ()
                      n310 = call "Delay T4.vi"("milliseconds to wait"=u32 10, "error in (no error)"=w1170) -> ("error out"=w1174:errorcluster)  [unwired: 9 in]
                      n311 = call "WS1050 AD7747 READ 36 DUT.vi"("error in"=w1174, "Log (T)"=w1167, "DUT Mask Mode (All)"=WSVCAP_SHL_I2C_DUT_Mask_Mode_Enum."C2") -> ("error out"=w1172:errorcluster, "AD7747 Values"=w1173:string[][])  [unwired: 7 in]
                      n312 = for {
                        tunnel: w1173 -> [w1186] mode=indexing
                        tunnel: w1172 -> [w1187]
                        tunnel: [w1187] -> w1168
                        tunnel: [w1184] -> w1176 mode=indexing
                        n313 = Index Array(array=w1186, index=3) -> (element=w1184:string)
                      }
                      n314 = Unbundle By Name(w1168) -> ("status"=w1182:bool)
                      n315 = Or(x=w1182, y=w1181) -> (x .or. y?=w1180:bool)
                    }
                  }
                  frame 1 {
                    n316 = for {
                      N: w1196 -> [_]
                      tunnel: w1194 -> [w1215]
                      tunnel: w1193 -> [w1213]
                      tunnel: [w1212] -> w1192
                      tunnel: [w1208] -> w1188 mode=indexing
                      tunnel: w1195 -> [w1210]
                      tunnel: w1190 -> [w1198]
                      tunnel: [w1200] -> w1191
                      tunnel: w1189 -> [w1199]
                      i -> [w1207]
                      stop <- w1212 stop-if-true
                      n317 = Index Array(array=w1215, index=w1207) -> (element=w1211:string)
                      n318 = Index Array(array=w1210, index=w1207) -> (element=w1209:string)
                      n319 = call "WSVCAP SHL Host TL RFFE Write - Multiple DUTs - Common Data.vi"("Data Out"=w1211, "error in"=w1198, "Log (T)"=FALSE) -> ("error out"=w1202:errorcluster)  [unwired: 12 in]
                      n320 = local write "STATUS"(w1209) -> ()
                      n321 = call "Delay T4.vi"("milliseconds to wait"=u32 10, "error in (no error)"=w1202) -> ("error out"=w1206:errorcluster)  [unwired: 9 in]
                      n322 = call "WS1050 AD7747 READ 36 DUT.vi"("error in"=w1206, "Log (T)"=w1199, "DUT Mask Mode (All)"=WSVCAP_SHL_I2C_DUT_Mask_Mode_Enum."C1") -> ("error out"=w1204:errorcluster, "AD7747 Values"=w1205:string[][])  [unwired: 7 in]
                      n323 = for {
                        tunnel: w1205 -> [w1218] mode=indexing
                        tunnel: w1204 -> [w1219]
                        tunnel: [w1219] -> w1200
                        tunnel: [w1216] -> w1208 mode=indexing
                        n324 = Index Array(array=w1218, index=1) -> (element=w1216:string)
                      }
                      n325 = Unbundle By Name(w1200) -> ("status"=w1214:bool)
                      n326 = Or(x=w1214, y=w1213) -> (x .or. y?=w1212:bool)
                    }
                  }
                }
                n327 = Transpose 2D Array(2D array=w1131) -> (transposed array=w1140:string[][])
                "40V_2" <- w1140
              }
              frame #3 {
                n328 = Array Size(array=w1239) -> (size(s)=w1240:i32)
                n329 = case shown="0, 1, Default" w1224 {
                  tunnel: w1240 -> [w1258 w1290]
                  tunnel: w1239 -> [w1257 w1289]
                  tunnel: w1238 -> [w1256 w1288]
                  tunnel: w1237 -> [w1255 w1287]
                  tunnel: [w1254 w1286] -> w1236
                  tunnel: w1231 -> [w1253 w1285]
                  tunnel: [w1252 w1284] -> w1223
                  tunnel: w1227 -> [w1251 w1283]
                  tunnel: [w1250 w1282] -> w1225
                  frame 0, 1, Default {
                    n330 = for {
                      N: w1258 -> [_]
                      tunnel: w1256 -> [w1277]
                      tunnel: w1255 -> [w1275]
                      tunnel: [w1274] -> w1254
                      tunnel: [w1270] -> w1250 mode=indexing
                      tunnel: w1257 -> [w1272]
                      tunnel: w1253 -> [w1260]
                      tunnel: [w1262] -> w1252
                      tunnel: w1251 -> [w1261]
                      i -> [w1269]
                      stop <- w1274 stop-if-true
                      n331 = Index Array(array=w1277, index=w1269) -> (element=w1273:string)
                      n332 = Index Array(array=w1272, index=w1269) -> (element=w1271:string)
                      n333 = local write "STATUS"(w1271) -> ()
                      n334 = call "WSVCAP SHL Host TL RFFE Write - Multiple DUTs - Common Data.vi"("Data Out"=w1273, "error in"=w1260, "Log (T)"=FALSE) -> ("error out"=w1264:errorcluster)  [unwired: 12 in]
                      n335 = call "Delay T4.vi"("milliseconds to wait"=u32 10, "error in (no error)"=w1264) -> ("error out"=w1268:errorcluster)  [unwired: 9 in]
                      n336 = call "WS1050 AD7747 READ 36 DUT.vi"("error in"=w1268, "Log (T)"=w1261, "DUT Mask Mode (All)"=WSVCAP_SHL_I2C_DUT_Mask_Mode_Enum."C3") -> ("error out"=w1266:errorcluster, "AD7747 Values"=w1267:string[][])  [unwired: 7 in]
                      n337 = for {
                        tunnel: w1267 -> [w1280] mode=indexing
                        tunnel: w1266 -> [w1281]
                        tunnel: [w1281] -> w1262
                        tunnel: [w1278] -> w1270 mode=indexing
                        n338 = Index Array(array=w1280, index=5) -> (element=w1278:string)
                      }
                      n339 = Unbundle By Name(w1262) -> ("status"=w1276:bool)
                      n340 = Or(x=w1276, y=w1275) -> (x .or. y?=w1274:bool)
                    }
                  }
                  frame 2 {
                    n341 = for {
                      N: w1290 -> [_]
                      tunnel: w1288 -> [w1309]
                      tunnel: w1287 -> [w1307]
                      tunnel: [w1306] -> w1286
                      tunnel: [w1302] -> w1282 mode=indexing
                      tunnel: w1289 -> [w1304]
                      tunnel: w1285 -> [w1292]
                      tunnel: [w1294] -> w1284
                      tunnel: w1283 -> [w1293]
                      i -> [w1301]
                      stop <- w1306 stop-if-true
                      n342 = Index Array(array=w1309, index=w1301) -> (element=w1305:string)
                      n343 = Index Array(array=w1304, index=w1301) -> (element=w1303:string)
                      n344 = local write "STATUS"(w1303) -> ()
                      n345 = call "WSVCAP SHL Host TL RFFE Write - Multiple DUTs - Common Data.vi"("Data Out"=w1305, "error in"=w1292, "Log (T)"=FALSE) -> ("error out"=w1296:errorcluster)  [unwired: 12 in]
                      n346 = call "Delay T4.vi"("milliseconds to wait"=u32 10, "error in (no error)"=w1296) -> ("error out"=w1300:errorcluster)  [unwired: 9 in]
                      n347 = call "WS1050 AD7747 READ 36 DUT.vi"("error in"=w1300, "Log (T)"=w1293, "DUT Mask Mode (All)"=WSVCAP_SHL_I2C_DUT_Mask_Mode_Enum."C1") -> ("error out"=w1298:errorcluster, "AD7747 Values"=w1299:string[][])  [unwired: 7 in]
                      n348 = for {
                        tunnel: w1299 -> [w1312] mode=indexing
                        tunnel: w1298 -> [w1313]
                        tunnel: [w1313] -> w1294
                        tunnel: [w1310] -> w1302 mode=indexing
                        n349 = Index Array(array=w1312, index=1) -> (element=w1310:string)
                      }
                      n350 = Unbundle By Name(w1294) -> ("status"=w1308:bool)
                      n351 = Or(x=w1308, y=w1307) -> (x .or. y?=w1306:bool)
                    }
                  }
                }
                n352 = Transpose 2D Array(2D array=w1225) -> (transposed array=w1232:string[][])
                "40V_3" <- w1232
              }
              frame #4 {
                # "VPI Testing @ 35V"
                n353 = call "WS1050 Delta C Calculation.vi"("error in (no error)"=w1355, "DCap Target(pF)"=w1354, "Input"=w1357) -> ("error out"=w1352:errorcluster, "Total Bank Delta C(pF)"=w1345:string[], "% Bank DeltaC"=w1349:string[])  [unwired: 4 in, 2 out]
                n354 = call "WS1050 Delta C Calculation.vi"("error in (no error)"=w1355, "DCap Target(pF)"=w1354, "Input"=w1356) -> ("error out"=w1353:errorcluster, "Total Bank Delta C(pF)"=w1344:string[], "% Bank DeltaC"=w1347:string[])  [unwired: 4 in, 2 out]
                n355 = call "WS1050 Delta C Calculation.vi"("error in (no error)"=w1355, "DCap Target(pF)"=w1354, "Input"=w1348) -> ("error out"=w1351:errorcluster, "Total Bank Delta C(pF)"=w1343:string[], "% Bank DeltaC"=w1346:string[])  [unwired: 4 in, 2 out]
                n356 = Merge Errors(w1352, w1353, w1351) -> (w1350:errorcluster)
                n357 = case shown="1, Default" w1358 {
                  tunnel: w1350 -> [w1388 w1396]
                  tunnel: [w1388 w1396] -> w1317
                  tunnel: w1349 -> [w1384 w1392]
                  tunnel: w1347 -> [w1383 w1391]
                  tunnel: w1346 -> [w1382 w1390]
                  tunnel: w1345 -> [w1387 w1395]
                  tunnel: [w1387 w1395] -> w1342
                  tunnel: w1344 -> [w1386 w1394]
                  tunnel: [w1386 w1394] -> w1341
                  tunnel: w1343 -> [w1385 w1393]
                  tunnel: [w1385 w1393] -> w1340
                  frame 0 {
                    n358 = Build Array(w1384, w1383, w1382) -> (→"% Delta C_T0":string[][])
                  }
                  frame 1, Default {
                    n359 = Build Array(w1392, w1391, w1390) -> (→"% Delta C":string[][])
                  }
                }
                "Total Delta C1(pF)" <- w1342
                "Total Delta C2(pF)" <- w1341
                "Total Delta C3(pF)" <- w1340
                n360 = call "WS1050_51 VPI Header.vi"("VPI Name"="VPI Name", "VPI_Cmd"="VPI_Cmd", "Cmin/Act"=w1315, "WS1050/51"=w1326, "error in (no error)"=w1327) -> ("VPI_1"=w1325:string[], "VPI_2"=w1323:string[], "VPI Header"=w1324:string[], "VPI_3"=w1322:string[], "Cmd_3"=w1319:string[], "Cmd_1"=w1321:string[], "Cmd_2"=w1320:string[], "error out"=w1318:errorcluster)  [unwired: 3 in]
                n361 = Merge Errors(w1318, w1317) -> (w1316:errorcluster)
                n362 = case shown="True" w1332 {
                  tunnel: w1372 -> [w1403 w1441]
                  tunnel: [w1399 w1419] -> w1336
                  tunnel: [w1397 w1443] -> w1371
                  tunnel: [w1397 w1427] -> w1370
                  tunnel: [w1403 w1425] -> w1368
                  tunnel: w1365 -> [w1405 w1442]
                  tunnel: [w1405 w1442] -> w1364
                  tunnel: w1321 -> [_ w1440]
                  tunnel: w1320 -> [_ w1434]
                  tunnel: w1319 -> [_ w1429]
                  tunnel: [w1397 w1439] -> w1361
                  tunnel: w1325 -> [w1402 w1437]
                  tunnel: w1323 -> [_ w1435]
                  tunnel: w1322 -> [_ w1430]
                  tunnel: ["" ("string") w1424] -> w1338
                  tunnel: w1316 -> [w1400 w1416]
                  frame False {
                    n363 = Array Size(array=w1402) -> (size(s)=w1401:i32)
                    n364 = for {
                      N: w1401 -> [_]
                      tunnel: [w1407] -> w1398 mode=indexing
                      tunnel: w1400 -> [w1406]
                      tunnel: [w1406] -> w1399
                      n365 = for {
                        N: 36 -> [_]
                        tunnel: [""] -> w1407 mode=indexing
                      }
                    }
                    n366 = Transpose 2D Array(2D array=w1398) -> (transposed array=w1397:string[][])
                    n367 = local write "VPI C1"(w1397) -> ()
                    n368 = local write "VPI C2"(w1397) -> ()
                    n369 = local write "VPI C3"(w1397) -> ()
                  }
                  frame True {
                    w1418 = FALSE ("Log (T)")
                    # "Set CP to 35V"
                    n370 = call "WSVCAP SHL Host TL RFFE Write - Multiple DUTs - Common Data.vi"("Data Out"="074820", "error in"=w1416, "Log (T)"=w1418) -> ("error out"=w1414:errorcluster)  [unwired: 12 in]
                    n371 = call "Delay T4.vi"("milliseconds to wait"=u32 10, "error in (no error)"=w1414) -> ("error out"=w1420:errorcluster)  [unwired: 9 in]
                    n372 = case shown="3" "CP VPI" {
                      selector: "CP VPI" -> [w1448 w1453 w1458 w1462]
                      tunnel: string[] ["07476F", "074776", "074765", "074769", "07477B"] -> [w1449 w1454 w1459 w1464]
                      tunnel: [w1447 w1452 w1457 w1463] -> w1412
                      tunnel: [w1445 w1450 w1455 w1460] -> w1411
                      tunnel: ["35" ("string") "27.5" ("string") "30.5" ("string") "40.25" ("string")] -> w1424
                      tunnel: w1420 -> [w1445 w1450 w1455 w1460]
                      frame 0, Default {
                        n373 = Index Array(array=w1449, index=w1448) -> (element=w1447:string)
                      }
                      frame 2 {
                        n374 = Index Array(array=w1454, index=w1453) -> (element=w1452:string)
                      }
                      frame 3 {
                        n375 = Index Array(array=w1459, index=w1458) -> (element=w1457:string)
                      }
                      frame 1 {
                        n376 = Index Array(array=w1464, index=w1462) -> (element=w1463:string)
                      }
                    }
                    n377 = Array Size(array=w1437) -> (size(s)=w1444:i32)
                    n378 = call "WSVCAP SHL Host TL RFFE Write - Multiple DUTs - Common Data.vi"("Data Out"=w1412, "error in"=w1411, "Log (T)"=w1418) -> ("error out"=w1423:errorcluster)  [unwired: 12 in]
                    n379 = for {
                      N: w1444 -> [_]
                      tunnel: w1440 -> [w1529]
                      tunnel: w1441 -> [w1527]
                      tunnel: [w1526] -> w1433
                      tunnel: [w1524] -> w1438 mode=indexing
                      tunnel: w1437 -> [w1523]
                      tunnel: w1423 -> [w1512]
                      tunnel: [w1514] -> w1422
                      i -> [w1522]
                      stop <- w1526 stop-if-true
                      n380 = Index Array(array=w1529, index=w1522) -> (element=w1525:string)
                      n381 = Index Array(array=w1523, index=w1522) -> (element=w1521:string)
                      n382 = local write "STATUS"(w1521) -> ()
                      n383 = call "WSVCAP SHL Host TL RFFE Write - Multiple DUTs - Common Data.vi"("Data Out"=w1525, "error in"=w1512, "Log (T)"=FALSE) -> ("error out"=w1520:errorcluster)  [unwired: 12 in]
                      n384 = call "Delay T4.vi"("milliseconds to wait"=u32 10, "error in (no error)"=w1520) -> ("error out"=w1516:errorcluster)  [unwired: 9 in]
                      n385 = call "WS1050 AD7747 READ 36 DUT.vi"("error in"=w1516, "Log (T)"=FALSE, "DUT Mask Mode (All)"=WSVCAP_SHL_I2C_DUT_Mask_Mode_Enum."C1") -> ("error out"=w1518:errorcluster, "AD7747 Values"=w1517:string[][])  [unwired: 7 in]
                      n386 = for {
                        tunnel: [w1532] -> w1524 mode=indexing
                        tunnel: w1518 -> [w1531]
                        tunnel: [w1531] -> w1514
                        tunnel: w1517 -> [w1530] mode=indexing
                        n387 = Index Array(array=w1530, index=1) -> (element=w1532:string)
                      }
                      n388 = Unbundle By Name(w1514) -> ("status"=w1528:bool)
                      n389 = Or(x=w1528, y=w1527) -> (x .or. y?=w1526:bool)
                    }
                    n390 = Transpose 2D Array(2D array=w1438) -> (transposed array=w1443:string[][])
                    "VPI C1" <- w1443
                    n391 = Array Size(array=w1435) -> (size(s)=w1436:i32)
                    n392 = for {
                      N: w1436 -> [_]
                      tunnel: w1434 -> [w1506]
                      tunnel: w1433 -> [w1504]
                      tunnel: [w1503] -> w1426
                      tunnel: [w1501] -> w1432 mode=indexing
                      tunnel: w1435 -> [w1500]
                      tunnel: w1422 -> [w1489]
                      tunnel: [w1491] -> w1421
                      i -> [w1499]
                      stop <- w1503 stop-if-true
                      n393 = Index Array(array=w1506, index=w1499) -> (element=w1502:string)
                      n394 = Index Array(array=w1500, index=w1499) -> (element=w1498:string)
                      n395 = call "WSVCAP SHL Host TL RFFE Write - Multiple DUTs - Common Data.vi"("Data Out"=w1502, "error in"=w1489, "Log (T)"=FALSE) -> ("error out"=w1497:errorcluster)  [unwired: 12 in]
                      n396 = local write "STATUS"(w1498) -> ()
                      n397 = call "Delay T4.vi"("milliseconds to wait"=u32 10, "error in (no error)"=w1497) -> ("error out"=w1493:errorcluster)  [unwired: 9 in]
                      n398 = call "WS1050 AD7747 READ 36 DUT.vi"("error in"=w1493, "Log (T)"=FALSE, "DUT Mask Mode (All)"=WSVCAP_SHL_I2C_DUT_Mask_Mode_Enum."C2") -> ("error out"=w1495:errorcluster, "AD7747 Values"=w1494:string[][])  [unwired: 7 in]
                      n399 = for {
                        tunnel: [w1509] -> w1501 mode=indexing
                        tunnel: w1495 -> [w1508]
                        tunnel: [w1508] -> w1491
                        tunnel: w1494 -> [w1507] mode=indexing
                        n400 = Index Array(array=w1507, index=3) -> (element=w1509:string)
                      }
                      n401 = Unbundle By Name(w1491) -> ("status"=w1505:bool)
                      n402 = Or(x=w1505, y=w1504) -> (x .or. y?=w1503:bool)
                    }
                    n403 = Transpose 2D Array(2D array=w1432) -> (transposed array=w1439:string[][])
                    "VPI C2" <- w1439
                    n404 = Array Size(array=w1430) -> (size(s)=w1431:i32)
                    n405 = for {
                      N: w1431 -> [_]
                      tunnel: w1429 -> [w1483]
                      tunnel: w1426 -> [w1481]
                      tunnel: [w1480] -> w1425
                      tunnel: [w1478] -> w1428 mode=indexing
                      tunnel: w1430 -> [w1477]
                      tunnel: w1421 -> [w1466]
                      tunnel: [w1468] -> w1419
                      i -> [w1476]
                      stop <- w1480 stop-if-true
                      n406 = Index Array(array=w1483, index=w1476) -> (element=w1479:string)
                      n407 = Index Array(array=w1477, index=w1476) -> (element=w1475:string)
                      n408 = call "WSVCAP SHL Host TL RFFE Write - Multiple DUTs - Common Data.vi"("Data Out"=w1479, "error in"=w1466, "Log (T)"=FALSE) -> ("error out"=w1474:errorcluster)  [unwired: 12 in]
                      n409 = local write "STATUS"(w1475) -> ()
                      n410 = call "Delay T4.vi"("milliseconds to wait"=u32 10, "error in (no error)"=w1474) -> ("error out"=w1470:errorcluster)  [unwired: 9 in]
                      n411 = call "WS1050 AD7747 READ 36 DUT.vi"("error in"=w1470, "Log (T)"=FALSE, "DUT Mask Mode (All)"=WSVCAP_SHL_I2C_DUT_Mask_Mode_Enum."C3") -> ("error out"=w1472:errorcluster, "AD7747 Values"=w1471:string[][])  [unwired: 7 in]
                      n412 = for {
                        tunnel: [w1486] -> w1478 mode=indexing
                        tunnel: w1472 -> [w1485]
                        tunnel: [w1485] -> w1468
                        tunnel: w1471 -> [w1484] mode=indexing
                        n413 = Index Array(array=w1484, index=5) -> (element=w1486:string)
                      }
                      n414 = Unbundle By Name(w1468) -> ("status"=w1482:bool)
                      n415 = Or(x=w1482, y=w1481) -> (x .or. y?=w1480:bool)
                    }
                    n416 = Transpose 2D Array(2D array=w1428) -> (transposed array=w1427:string[][])
                    "VPI C3" <- w1427
                  }
                }
                n417 = Insert Into Array(array=w1360, new element=w1324) -> (w1359:string[])  [unwired: 1 in]
                n418 = case shown="True" w1337 {
                  tunnel: w1336 -> [w1374 w1379]
                  tunnel: [w1375 w1378] -> w1335
                  frame False {
                    n419 = call "WSVCAP SHL Host TL RFFE Write - Multiple DUTs - Common Data.vi"("Data Out"="074820", "error in"=w1374, "Log (T)"=FALSE) -> ("error out"=w1375:errorcluster)  [unwired: 12 in]
                  }
                  frame True {
                    n420 = call "WSVCAP SHL Host TL RFFE Write - Multiple DUTs - Common Data.vi"("Data Out"="074800", "error in"=w1379, "Log (T)"=FALSE) -> ("error out"=w1378:errorcluster)  [unwired: 12 in]
                  }
                }
                n421 = call "Delay T4.vi"("milliseconds to wait"=u32 10, "error in (no error)"=w1335) -> ("error out"=w1334:errorcluster)  [unwired: 9 in]
              }
              frame #5 {
                # "VSA Testing"
                n422 = case shown="False" w1535 {
                  tunnel: w1574 -> [w1586 w1600]
                  tunnel: [w1585 w1599] -> w1548
                  tunnel: [w1590 w1606] -> w1564
                  tunnel: w1565 -> [w1590 w1605]
                  tunnel: [w1587 w1603] -> w1553
                  tunnel: [w1587 w1602] -> w1550
                  tunnel: [w1587 w1601] -> w1547
                  tunnel: [w1588 w1604] -> w1554
                  frame False {
                    n423 = for {
                      tunnel: dbl[] [0.0, 0.0, 0.0] -> [w1595] mode=indexing
                      tunnel: [w1594] -> w1588 mode=indexing
                      tunnel: [w1592] -> w1587 mode=indexing
                      tunnel: w1586 -> [w1591]
                      tunnel: [w1591] -> w1585
                      w1593 = 36
                      n424 = Number To Fractional String(number=w1595) -> (F-format string=w1596:string)  [unwired: 3 in]
                      n425 = for {
                        N: w1593 -> [_]
                        tunnel: w1596 -> [w1598]
                        tunnel: [w1598] -> w1594 mode=indexing
                      }
                      n426 = for {
                        N: w1593 -> [_]
                        tunnel: [""] -> w1592 mode=indexing
                      }
                    }
                  }
                  frame True {
                    n427 = for {
                      tunnel: "VSA Voltage(V)" -> [w1630] mode=indexing
                      tunnel: [w1634] -> w1606
                      tunnel: w1605 -> [w1632]
                      tunnel: [w1631] -> w1603 mode=indexing
                      tunnel: [w1618] -> w1602 mode=indexing
                      tunnel: [w1627] -> w1604 mode=indexing
                      tunnel: [w1612] -> w1601 mode=indexing
                      tunnel: w1600 -> [w1611]
                      tunnel: [w1610] -> w1599
                      w1609 = FALSE ("Log (T)")
                      w1626 = u16 0 items=["Voltage", "Current"] ("Source Mode  (0: Voltage)")
                      n428 = call "Ke2400 Configure Output.vi"("Source Mode  (0: Voltage)"=w1626, "error in (no error)"=w1611, "Compliance  Level (0.1)"=0.1, "Output Level (0)"=w1630, "VISA resource name"=w1632) -> ("error out"=w1638:errorcluster, "VISA resource name out"=w1636:refnum<visa-resource-name>)  [unwired: 5 in]
                      n429 = Number To Fractional String(number=w1630) -> (F-format string=w1629:string)  [unwired: 3 in]
                      n430 = call "Ke2400 Enable.vi"("error in (no error)"=w1638, "ON/OFF"=TRUE ("Enable Output (T: Enable)"), "VISA resource name"=w1636) -> ("error out"=w1639:errorcluster, "VISA resource name out"=w1634:refnum<visa-resource-name>)  [unwired: 7 in]
                      n431 = call "Delay T4.vi"("milliseconds to wait"=u32 10, "error in (no error)"=w1639) -> ("error out"=w1625:errorcluster)  [unwired: 9 in]
                      n432 = call "WS1050 AD7747 READ 36 DUT.vi"("error in"=w1625, "Log (T)"=w1609, "DUT Mask Mode (All)"=WSVCAP_SHL_I2C_DUT_Mask_Mode_Enum."C1") -> ("error out"=w1622:errorcluster, "AD7747 Values"=w1624:string[][])  [unwired: 7 in]
                      n433 = for {
                        tunnel: w1624 -> [w1650] mode=indexing
                        tunnel: [w1651] -> w1631 mode=indexing
                        tunnel: w1622 -> [w1649]
                        tunnel: [w1649] -> w1621
                        n434 = Index Array(array=w1650, index=1) -> (element=w1651:string)
                      }
                      n435 = for {
                        N: 36 -> [_]
                        tunnel: w1629 -> [w1648]
                        tunnel: [w1648] -> w1627 mode=indexing
                      }
                      n436 = call "WS1050 AD7747 READ 36 DUT.vi"("error in"=w1621, "Log (T)"=w1609, "DUT Mask Mode (All)"=WSVCAP_SHL_I2C_DUT_Mask_Mode_Enum."C2") -> ("error out"=w1619:errorcluster, "AD7747 Values"=w1617:string[][])  [unwired: 7 in]
                      n437 = for {
                        tunnel: w1617 -> [w1645] mode=indexing
                        tunnel: [w1646] -> w1618 mode=indexing
                        tunnel: w1619 -> [w1644]
                        tunnel: [w1644] -> w1616
                        n438 = Index Array(array=w1645, index=3) -> (element=w1646:string)
                      }
                      n439 = call "WS1050 AD7747 READ 36 DUT.vi"("error in"=w1616, "Log (T)"=w1609, "DUT Mask Mode (All)"=WSVCAP_SHL_I2C_DUT_Mask_Mode_Enum."C3") -> ("error out"=w1614:errorcluster, "AD7747 Values"=w1613:string[][])  [unwired: 7 in]
                      n440 = for {
                        tunnel: w1613 -> [w1641] mode=indexing
                        tunnel: [w1642] -> w1612 mode=indexing
                        tunnel: w1614 -> [w1640]
                        tunnel: [w1640] -> w1610
                        n441 = Index Array(array=w1641, index=5) -> (element=w1642:string)
                      }
                    }
                    n442 = local write "STATUS"("VSA Testing...." ("STATUS")) -> ()
                  }
                }
                n443 = Transpose 2D Array(2D array=w1554) -> (transposed array=w1552:string[][])
                n444 = Transpose 2D Array(2D array=w1553) -> (transposed array=w1551:string[][])
                n445 = Transpose 2D Array(2D array=w1550) -> (transposed array=w1549:string[][])
                n446 = Transpose 2D Array(2D array=w1547) -> (transposed array=w1546:string[][])
                n447 = call "WS1050_VSA_Convert_Data.vi"("VSA_C3"=w1546, "error in (no error)"=w1548, "VSA_C2"=w1549, "VSA_C1"=w1551, "Voltage"=w1552) -> ("error out"=w1545:errorcluster, "VSA_V3"=w1542:string[][], "VSA_V2"=w1543:string[][], "VSA_V1"=w1544:string[][])  [unwired: 3 in]
                "VSA_V1" <- w1544
                "VSA_V2" <- w1543
                "VSA_V3" <- w1542
                n448 = case shown="True" w1535 {
                  tunnel: w1564 -> [w1578 w1584]
                  tunnel: [w1578 w1583] -> w1563
                  tunnel: w1545 -> [w1577 w1582]
                  tunnel: [w1577 w1579] -> w1562
                  frame False {
                  }
                  frame True {
                    w1580 = u16 0 items=["Voltage", "Current"] ("Source Mode  (0: Voltage)")
                    n449 = call "Ke2400 Configure Output.vi"("Source Mode  (0: Voltage)"=w1580, "error in (no error)"=w1582, "Output Level (0)"=0.0, "VISA resource name"=w1584) -> ("error out"=w1579:errorcluster, "VISA resource name out"=w1583:refnum<visa-resource-name>)  [unwired: 6 in]
                  }
                }
                n450 = call "Delay T4.vi"("milliseconds to wait"=u32 50, "error in (no error)"=w1562) -> ("error out"=w1561:errorcluster)  [unwired: 9 in]
              }
              frame #6 {
                # "Handshake Check and EFuse Readback"
                n451 = Or(x=w1662, y=w1672) -> (x .or. y?=w1671:bool)
                n452 = Add(x=w1684, y=w1683) -> (x+y=w1670:u64)
                n453 = case shown="True" w1671 {
                  tunnel: w1697 -> [w1710 _]
                  tunnel: w1696 -> [w1709 w1715]
                  tunnel: [w1708 w1715] -> w1695
                  tunnel: w1694 -> [w1707 _]
                  tunnel: w1693 -> [w1706 _]
                  tunnel: w1692 -> [w1705 _]
                  tunnel: [w1701 w1714] -> w1691
                  tunnel: [w1700 w1714] -> w1686
                  tunnel: w1670 -> [w1699 _]
                  tunnel: w1677 -> [w1698 _]
                  frame False {
                    n454 = call "WS1050_36DUT_Handshake Check R1_Record All Regs Ver1.0.vi"("file path (use dialog)"=w1710, "Reg1_Bit Cntrl"="Reg1_Bit Cntrl", "File Name"=w1698, "SN"=w1705, "Loop"=w1699, "error"=w1709, "Lot #"=w1707, "Wafer #"=w1706) -> ("Pass/Fail"=→"EFuse Readback Status":bool[], "EFuse Read back"=w1700:string[], "Status"=w1701:string[], "error out"=w1708:errorcluster)  [unwired: 6 in, 2 out]
                    n455 = case shown="1, Default" w1699 {
                      tunnel: w1700 -> [w1711 w1712]
                      frame 0 {
                        "EFuse RB T0" <- w1711
                      }
                      frame 1, Default {
                        "Current EFuse Read back" <- w1712
                      }
                    }
                    n456 = local write "STATUS"("Hand Shake & EFuse Readback...." ("STATUS")) -> ()
                  }
                  frame True {
                    n457 = for {
                      N: 36 -> [_]
                      tunnel: [""] -> w1714 mode=indexing
                    }
                  }
                }
                n458 = Add(x=w1670, y=w1667) -> (x+y=w1668:u64)
                "TTCompleted" <- w1668
                n459 = Number To Engineering String(4:w1668) -> (0:w1682:string)  [unwired: 3 in]
                n460 = Build Array(w1681, w1679, w1678) -> (w1680:string[])
              }
              frame #7 {
                # "Save Data"
                n461 = Increment(x=w1728) -> (x+1=w1727:i32)
                n462 = local write "STATUS"("Saving Data...." ("STATUS")) -> ()
                n463 = Multiply(x=w1727, y=36) -> (x*y=w1722:i32)
                n464 = Path To String(path=w1732) -> (string=w1731:string)
                n465 = Bundle("Test Program"=w1764, "Comment"=w1763, "Data Out"=w1739, "Data Out"=w1738, "CP Voltage"=w1737, w1736, "Data Out"=w1735, "CP Voltage"=w1734, "string"=w1733, "Freq(Hz)"=w1720, "Board#"=w1718) -> (w1719:T8)  [unwired: 1 in]
                n466 = case shown="True" "Debug" {
                  tunnel: w1722 -> [w1771 w1774]
                  tunnel: [w1771 w1772] -> w1721
                  frame False {
                  }
                  frame True {
                    n467 = Multiply(x=w1774, y="No of Rows\nFrom Spread Sheet") -> (x*y=w1772:i32)
                  }
                }
                n468 = call "WS1050_36 DUT SData Ver1.0.vi"("TMN DC\\CAP Data Log File Path"=w1732, "Lot#"=w1766, "Total Delta C1(pF)"=w1742, "VSA_V1"=w1751, "Wafer#"=w1762, "File Name"=w1725, "Total Delta C2(pF)"=w1741, "error in"=w1769, "TP/Comment"=w1719, "EFuse"=w1756, "Data Output C3"=w1744, "Temperature"=w1748, "VSA_V2"=w1752, "VPI C3"=w1746, "Data Output C1"=w1759, "VPI C2"=w1745, "SN"=w1767, "R/W Status"=w1765, "Cap Header"=w1747, "HD/Cycles Completed"=w1755, "Data Output C2"=w1743, "VSA_V3"=w1750, "Current"=w1758, "VPI C1"=w1757, "Total Delta C3(pF)"=w1740) -> ("error out"=w1768:errorcluster)  [unwired: 2 in]
                n469 = Concatenate Strings(w1731, "\\" ("string"), w1725, "_Multi Socket Data.csv" ("string")) -> (w1730:string)
              }
              frame #8 {
                n470 = case shown="True" "Plot Delta Cmin" {
                  tunnel: w1781 -> [w1794 w1809]
                  tunnel: [w1794 w1805] -> w1780
                  tunnel: w1779 -> [_ w1801]
                  tunnel: w1777 -> [_ w1799]
                  frame False {
                  }
                  frame True {
                    n471 = String To Path(string=w1801) -> (path=w1800:path)
                    n472 = call "Delay T4.vi"("milliseconds to wait"=u32 50, "error in (no error)"=w1809) -> ("error out"=w1808:errorcluster)  [unwired: 9 in]
                    n473 = call "36DUT Plot From Spread Sheet.vi"("Plot"="Plot", "No of Rows"=w1799, "error in (no error)"=w1808, "Bank"="Bank", "file path (dialog if empty)"=w1800) -> ("error out"=w1803:errorcluster, "Delta C_Min Plot"=→"Plot_1":dbl[][])  [unwired: 5 in]
                    n474 = call "36DUT Plot From Spread Sheet.vi"("Plot"="Plot", "No of Rows"=w1799, "error in (no error)"=w1803, "Bank"="Bank 2", "file path (dialog if empty)"=w1800) -> ("error out"=w1804:errorcluster, "Delta C_Min Plot"=→"Plot_2":dbl[][])  [unwired: 5 in]
                    n475 = call "36DUT Plot From Spread Sheet.vi"("Plot"="Plot", "No of Rows"=w1799, "error in (no error)"=w1804, "Bank"="Bank 3", "file path (dialog if empty)"=w1800) -> ("error out"=w1805:errorcluster, "Delta C_Min Plot"=→"Plot_3":dbl[][])  [unwired: 5 in]
                  }
                }
                n476 = Get Date/Time In Seconds() -> (seconds since 1Jan1904=w1787:timestamp)
                n477 = Get Date/Time String(seconds (now)=w1787, want seconds? (F)=TRUE) -> (date string=→"date string":string, time string=→"Previous Time":string)  [unwired: 1 in]
                n478 = local write "RB Reg for HD/Cycle"(string[] []) -> ()
                n479 = Greater Or Equal?(x=w1784, y=w1776) -> (x >= y?=w1791:bool)
                n480 = Greater Or Equal?(x=w1783, y=w1776) -> (x >= y?=w1782:bool)
                "No of HD/Cycle\nCompleted" <- w1784
              }
            }
            n481 = Increment(x=w590) -> (x+1=→"Loop \ncompleted":i32)
            n482 = call "Delay T4.vi"("milliseconds to wait"=u32 10, "error in (no error)"=w484) -> ("error out"=w485:errorcluster)  [unwired: 9 in]
            n483 = Compound Arithmetic op=OR(w658, w561, w586) -> (w599:bool)
          }
          "Total Time" <- w409
          n484 = Increment(x=w407) -> (x+1=→"Run Loops":i32)
          n485 = local write "No of HD/Cycle\nCompleted"(u64 0 ("No of HD/Cycle\nCompleted")) -> ()
          n486 = Unbundle By Name(w399) -> ("status"=w413:bool)
          n487 = Compound Arithmetic op=OR(w413, w405, w404) -> (w395:bool)
        }
        n488 = for {
          tunnel: w291 -> [w1821]
          tunnel: w269 -> [w1820]
          tunnel: w320 -> [w1818] mode=indexing
          tunnel: [w1813] -> w289
          tunnel: [w1817] -> w319
          n489 = call "E3631A_Voltage Controller updated.vi"("VISA resource name"=w1820, "I_VDD(A)"=0.5, "Channel Controller"=w1818, "Voltage 1"=0.0, "Voltage 2"=3.3, "error in (no error)"=w1821, "I_3.3V (A)"=0.5) -> ("VISA resource name out"=w1817:refnum<visa-resource-name>, "error out"=w1814:errorcluster)  [unwired: 7 in]
          n490 = call "Delay T4.vi"("milliseconds to wait"=u32 100, "error in (no error)"=w1814) -> ("error out"=w1813:errorcluster)  [unwired: 9 in]
        }
        n491 = VISA Write(VISA resource name=w310, write buffer="SOUR:FUNC VOLT;VOLT:MODE FIX;RANG 100;LEV 0.0;:SENS:FUNC \"CURR\";CURR:PROT 60E-3;RANG 100E-3;:OUTP ON", error in (no error)=w291) -> (VISA resource name out=w308:refnum<visa-resource-name>, error out=w290:errorcluster)  [unwired: 1 out]
        n492 = Merge Errors(w289, w290) -> (w309:errorcluster)
      }
      frame True {
      }
    }
    n493 = local write "stop During HD/Cycles"(w70) -> ()
    n494 = Wait Until Next ms Multiple(millisecond multiple=u32 100) -> ()  [unwired: 1 out]
    n495 = Unbundle By Name(w71) -> ("status"=w89:bool)
    n496 = Or(x=w89, y=w80) -> (x .or. y?=w88:bool)
    "STATUS" <- "Idle...." ("STATUS")
  }
  "Ke2000 Out" <- w22
  "PS1 Out" <- w21
  n497 = local write "stop During HD/Cycles"(w7) -> ()
  n498 = local write "stop"(w7) -> ()
  n499 = case shown="True" w19 {
    tunnel: [w1838 w1841] -> w2
    tunnel: w13 -> [w1838 w1840]
    frame False {
    }
    frame True {
      n500 = local write "Online"(FALSE ("Online")) -> ()
      n501 = call "WSVCAP SHL Host TL Close.vi"("error in"=w1840) -> ("error out"=w1841:errorcluster)  [unwired: 14 in]
    }
  }
  "error out" <- w2
  n502 = VISA Write(VISA resource name=w14, write buffer="SOUR:FUNC VOLT;VOLT:MODE FIX;RANG 100;LEV 0.0;:SENS:FUNC \"CURR\";CURR:PROT 60E-3;RANG 100E-3;:OUTP OFF", error in (no error)=w13) -> (VISA resource name out=→"VISA resource name out":refnum<visa-resource-name>, error out=→"error out 2":errorcluster)  [unwired: 1 out]
